vi "UHR-Fleezers Control (fpga) - avogadro 7b enable apd ct.vi"() -> ()   [LabVIEW 2014]
doc: "UHR-Fleezers Instrument Control Code (fpga)"
uses:
  <vilib>/Platform/TimedLoop/XDataNode/timing_clust.ctl
  <vilib>/Platform/TimedLoop/XDataNode/nitl_modes.ctl
  <vilib>/Platform/TimedLoop/XDataNode/wakeup.ctl
  <vilib>/rvi/Emulation/niFpgaGetClockAttributes.vi
  <vilib>/rvi/Emulation/niFpgaSctlEmulationGetInTimedLoop.vi
  <vilib>/rvi/Emulation/niFpgaEmulationReportErrorSimple.vi
  <vilib>/rvi/Emulation/niFpgaProcessEmulError.vi
  <vilib>/rvi/eio/common/nirviEmuTemplateMethod_errors.vi
  <vilib>/rvi/Emulation/niFpgaCriticalErrorInLSC.vi
  <vilib>/rvi/interface/RandomDataEmulation/niFpgaRandomDataHandleErrors.vi
  <vilib>/rvi/Emulation/niFpgaEmulationIsFPGAContextNoSignature.vi
  <vilib>/rvi/errors/niFpgaSetErrorForExecOnDevCompSimple.vi
  <vilib>/rvi/eio/common/nirviEmuReportErrorAndStop.vi
  <vilib>/rvi/DataTransferAndStorage/Container/Common/niFpgaContainerGetUniqueNameForEmu.vi
  <vilib>/rvi/FIFO/Fifo_Resource/nirvififoEmulationSetSize.vi
  <vilib>/rvi/FIFO/Fifo_Resource/nirviFifoEmulationQueueMgr.vi
  <instcachedir>/0/nirviFifoEmulationQueueMgr_E5CAEC123FF24DC58D834DCA3CDAA9B5.lvgen/nirviFifoEmulationQueueMgr_E5CAEC123FF24DC58D834DCA3CDAA9B5_001.vi
  <vilib>/rvi/FIFO/Fifo_Resource/nirvififoEmulationDetermineInputValidOut.vi
  <vilib>/rvi/FIFO/Fifo_Resource/nirvififoEmulationCreateLock.vi
  <vilib>/rvi/FIFO/Fifo_Resource/nirvififoEmulationObtainLock.vi
  <vilib>/rvi/FIFO/Fifo_Resource/nirvififoEmulationReleaseLock.vi
  <vilib>/rvi/occurrence/nirviWaitOnOccurrenceBase.vi
  <vilib>/rvi/errors/nirviReportUnexpectedCaseInternalError.vi
  <vilib>/rvi/errors/nirviReportUnexpectedCaseInternalError (U32).vi
  <vilib>/rvi/DataTransferAndStorage/Container/Common/niFpgaContainerExecOnDevCompGetState.vi
  <vilib>/Utility/error.llb/Clear Errors.vi
  <vilib>/eio/EIONode/EIONode.xnode
  <vilib>/eio/EIOMethodNode/EIOMethodNode.xnode
  <vilib>/rvi/DataTransferAndStorage/Container/XNode/niFpgaContainer.xnode
  <vilib>/rvi/interface/RandomDataEmulation/nirviRandomDataFpgaReadWriteTemplate.vi
  <vilib>/rvi/FIFO/Fifo_Resource/nirvififoEmulationWrite.vi
  <vilib>/rvi/FIFO/Fifo_Resource/niFpgaFifoEmulationRefIn.vi
  <vilib>/addons/control/pid/fpga.llb/XNode/niFpgaPID.xnode
  <vilib>/Platform/TimedLoop/XDataNode/XDataNode.xnode
  <vilib>/rvi/FIFO/Fifo_Resource/nirvififoEmulationRead.vi
  <vilib>/Platform/TimedLoop/XDataNode/XDNodeRunTimeDep.lvlib
  <vilib>/rvi/Memory/Memory_Emulation/niFpgaMemoryEmulationRefIn.vi
panel:
  in  "BD 1 Delay (ticks)":u8
  out "lifetime (ticks)":u16
  in  "Lifetime to FIFO":bool
  in  "Tab Control":T1(tab)=enum."MCL trap control"
  in  "Set 3":bool
  in  "Set 2":bool=TRUE
  in  "Set 1":bool=TRUE
  in  "Trap Pos to FIFO":bool
  in  "N of AI1 Int Acq Sets":i16=2 min=1 max=3 step=1
  out "AI Late Counter":u8
  in  "ai count":u16=400
  in  "+ phase":bool
  in  "Phase count adjustment":i16
  out "Relative phase":i16
  in  "AI to FIFO":bool
  out "BD1 Frequency Out 1":u64
  out "BD1 Frequency Out 2":u64
  out "Trap Pos FIFO Timeout":u16
  out "Trap AI FIFO Timeout":u16
  in  "Trap FIFO Set Timeout":i32
  in  "Tab Control 2":T2(tab)
  in  "Multiple trap 3 position offset \nfile":bool
  in  "Piezo offset Y points":u64
  in  "Piezo offset X points":u64
  in  "Piezo offset Xmin":u64
  in  "Piezo Offset Ymin":u64
  in  "Piezo Offset Increment":u64
  out "BD1 amplitude 1 out":u16
  out "BD1 amplitude 2 out":u16
  in  "FB output range":cluster{"output low":i16, "output high":i16}={"output low"=0, "output high"=3000}
  in  "FB Gains":T3={"proportional gain (Kc)"=10, "integral gain (Kc*Ts/Ti)"=5, "derivative gain (Kc*Td/Ts)"=0}
  in  "RF synth green feedback max":i16=4000
  in  "RD":bool=TRUE
  in  "Swap F1 and F2":bool
  in  "Cont. Scan":bool
  in  "Abort scan":bool
  in  "Cycles per step":u64
  in  "Scan BD":bool
  in  "Number of scans":u16
  in  "Scan steps":u64
  in  "Scan freq.  increment":i64
  out "Scanning":bool
  in  "Start scan":bool
  in  "OSK Bd 1":bool
  in  "Reset Bd 1":bool
  in  "PMODE":bool=TRUE
  in  "Number Interlace Cycles":u8=2 min=1 max=3
  in  "Interlace Off Parameters":u8=1 min=1 max=3
  in  "Interlace ON/OFF":bool
  out "DIO Relative phase":i16
  in  "Phase count adjustment (DIO)":i16
  in  "+ phase (DIO)":bool
  out "DIO Late Counter":u8
  in  "DIO count 1 (ticks)":u16=400
  in  "DIO count 2 (ticks)":u16=400
  in  "DIO count 3 (ticks)":u16=400
  out "AI2 Y Sum Set 2":i16
  out "AI2 Y Sum Set 1":i16
  in  "FB Setpoint Set 1":i16 min=0 step=1
  in  "FB Reset Set 1":bool
  in  "FB On/Off Set 1":bool
  in  "FB Reset Set 2":bool
  in  "FB On/Off Set 2":bool
  in  "FB Setpoint Set 2":i16 min=0 step=1
  out "Scan I":u64
  in  "Amp switch delay":u8=5
  in  "RF synth bd controls green":bool
  in  "Phase Trap 2":fxp<+,14,14>
  in  "Phase Trap 1":fxp<+,14,14>
  in  "Phase offset method":u8
  in  "BD 1 Amplitude 1":u16
  in  "BD 1 Frequency 1":u64
  in  "BD 1 Amplitude 2":u16
  in  "BD 1 Frequency 2":u64
  in  "BD 1 Amplitude 3":u16
  in  "BD 1 Frequency 3":u64
  in  "Next trap write delay (ticks)":u8 caption="Count(Ticks)"
  out "Random phase generated":fxp<+,14,14>
  in  "RF phase reset before cycles":bool
  in  "Ready Write":bool
  in  "Data":i64
  in  "Address 2":u32
  out "Piezo X out":i16
  out "Piezo Y out":i16
  in  "Piezo Trap ON/Off (AO3)":i16
  in  "Piezo Trap X (AO5)":i16
  in  "Piezo Trap Y (AO4)":i16
  in  "Symmetric force feedback\nand raster scan":bool
  in  "FB Min frequency":u64
  in  "FB Max Frequency":u64
  in  "Dynamic Force FB (Ronen)":bool
  in  "Trap pos. FB Range":T4={"FB2 output low"=-1.0, "FB2 output high"=0.999969482421875}
  in  "Trap Pos. FB Gains":T5={"proportional gain (Kc)"=0.999969482421875, "integral gain (Kc*Ts/Ti)"=0.999969482421875, "derivative gain (Kc*Td/Ts)"=0.0}
  in  "B factor":fxp<+/-,32,16>
  in  "Negate Diff?":bool
  in  "Diff FB Measurement?":bool
  in  "FB Trig Integrate":u32=1
  out "TTrig?":bool
  in  "TTrig Negate Pos":bool=TRUE
  out "Trap Pos FB Int Signal":fxp<+/-,24,9> format="%.18g"
  out "Trap Pos FB Int-Norm Signal":fxp<+/-,16,1> format="%.16g"
  in  "FPGA TTrig Thresh":i64
  in  "FPGA Trap Trig":bool
  out "Trap Pos FB Action":i64
  in  "Trap Pos. FB Offset Factor":i64
  in  "Trap Pos. FB Mult Factor":i64=2
  in  "Trap Pos. FB Reset":bool
  in  "Trap Pos FB Monitor T1 or T2":bool
  in  "AI1 X Scale":u16
  in  "Trap Pos FB Int Count":u16=100
  in  "Trap Pos FB Negate Action":bool
  out "AI1 X Set 2":fxp<+/-,16,1>
  out "AI1 X Set 1":fxp<+/-,16,1>
  in  "Trap Pos. FB SP":fxp<+/-,16,1>
  in  "Force feedback":bool
  out "TTrig Sig":i64
  out "TTrig Fin Thresh":i64
  in  "ScanTrap 3 or Fl-laser":bool
  in  "1D or 2D Scan?":bool
  in  "Abort scan (MCL)":bool
  in  "MCL Scan Axis":bool
  in  "Cont. Scan (MCL)":bool
  out "Scan I (MCL)":u64
  in  "Number of scans (MCL)":u16
  out "Scanning MCL":bool
  in  "Scan steps (MCL)":u64
  in  "Cycles per step (MCL)":u64
  in  "Scan freq.  increment (MCL)":i16
  in  "Start scan (MCL)":bool
  in  "AO2 (X)":i16
  in  "AO1 (Y)":i16
  out "MCL Late Counter":u8
  in  "MCL count":u32=800
  out "MCL Relative Phase":i16
  in  "Phase count adjustment (MCL)":i16
  in  "+ phase (MCL)":bool
  in  "Lifetime events to read blue":u16=100
  in  "Lifetime read blue fifo":bool
  out "lifetime events in fifo":u16
  out "APD2 int gate":bool
  out "APD3 out state":bool
  in  "APD Gate Operating Mode":u8 max=2 step=1
  in  "Invert APD Gate":bool
  in  "APD Gate OFF Count":u16=100
  in  "APD Gate ON Count":u16=300
  out "APD 1 Gate Late Counter":u8
  out "APD 1 Gate Relative Phase":i16
  in  "Phase count adjustment (APD 1 Gate)":i16
  in  "+ phase (APD 1 Gate)":bool
  out "APD 2 Counts 0":u32
  out "APD 2 Counts 1":u32
  out "APD 1 Counts 0":u32
  out "APD 1 Counts 1":u32
  out "APD1 out state":bool
  in  "APD AO scale factor":i16=1
  in  "APD to FIFO":bool
  in  "APD Acq Rate Count":u32=20000000
  out "APD Acq Late Counter":u8
  out "APD Acq Relative Phase":i16
  in  "Phase Count Adjustment (APD Acq)":i16
  in  "+ phase (APD Acq)":bool
  in  "Phase count adjustment (APD 2 Gate)":i16
  out "APD 2 Gate Late Counter":u8
  out "APD 2 Gate Relative Phase":i16
  in  "+ phase (APD 2 Gate)":bool
  out "APD2 out state":bool
  out "APD 3 Counts 0":u32
  out "APD 3 Counts 1":u32
  out "APD 3 Gate Late Counter":u8
  in  "Phase count adjustment (APD 3 Gate)":i16
  out "APD 3 Gate Relative Phase":i16
  in  "+ phase (APD 3 Gate)":bool
  out "APD1 int gate":bool
  out "APD3 int gate":bool
  in  "Lifetime timeout APD1":u16=200
  in  "Laser choice 2":u8=100
  in  "Laser choice 1":u8=100
  in  "Laser choice 0":u8=100
  in  "FL interlace OFF count 2":u16=100
  in  "FL interlace OFF count 1":u16=100
  in  "FL interlace ON count 2":u16=300
  in  "Fl interlace ON count 1":u16=300
  in  "D3 2":i16
  in  "I3 2":i16=5
  in  "P3 2":i16=10
  in  "Green FB Setpoint 2":i16=250 min=0 step=1
  in  "Green FB Reset 2":bool
  in  "D3":i16
  in  "I3":i16=5
  in  "P3":i16=10
  in  "Green Filter Flipper":bool
  in  "Green FB Count":u16=1200
  out "Green Late Counter":u8
  out "Green FB Relative Phase":i16
  in  "Phase count adjustment (Green FB)":i16=10
  in  "+ phase (Green FB)":bool
  out "Green FB Sum":i16
  in  "Green int current ON count adj":u16=150
  in  "Current Out":u16=30000
  in  "Green FB On/Off":bool
  in  "Green FB Setpoint":i16=250 min=0 step=1
  in  "Green FB Reset":bool
  in  "Operating Mode 2":u8=2 max=2 step=1
  in  "Invert GI 2":bool
  in  "Green interlace OFF count 2":u16=900
  in  "Green interlace ON count 2":u16=300
  out "GI Late Counter 2":u8
  out "GI Relative phase 2":i16
  in  "Phase count adjustment (GI) 2":i16=20
  in  "+ phase (GI) 2":bool
  in  "FL interlace OFF count 0":u16=100
  out "GI Relative phase":i16
  in  "Phase count adjustment (GI)":i16
  in  "+ phase (GI)":bool
  in  "FL interlace ON count 0":u16=300
  out "GI Late Counter":u8
  in  "Invert GI":bool
  in  "Operating Mode":u8 max=2 step=1
  out "green FB running":bool
  in  "+ phase (RI)":bool
  out "RI Relative phase":i16
  out "RI Late Counter":u8
  in  "Red interlace ON count":u16=300
  in  "Red interlace OFF count":u16=100
  in  "Invert RI":bool
  in  "Red Laser Operating Mode":u8 max=2 step=1
  in  "Phase count adjustment (RI)":i16
  out "Red FB Intensity":i16
  in  "RI Current Out":u16=30000
  in  "Red FB On/Off":bool
  in  "D4":i16
  in  "I4":i16=5
  in  "P4":i16=10
  in  "Red FB Setpoint":i16=250 min=0 step=1
  in  "Red FB Reset":bool
  in  "RI Operating Mode 2":u8=2 max=2 step=1
  in  "Invert RI 2":bool
  in  "Phase count adjustment (BI AO)":i16=20
  in  "Blue current ON count adj (AO)":u16=150
  in  "BI Current Out":i16=30000
  in  "Blue FB On/Off":bool
  in  "D5":i16
  in  "I5":i16=5
  in  "P5":i16=10
  in  "Blue FB Setpoint":i16=250 min=0 step=1
  in  "Blue FB Reset":bool
  in  "BI Operating Mode (AO)":u8=2 max=2 step=1
  in  "Invert BI (AO)":bool
  in  "Blue OFF count (AO)":u16=900
  in  "Blue ON count (AO)":u16=300
  out "BI Late Counter (AO)":u8
  out "BI Relative phase (AO)":i16
  in  "+ phase (BI AO)":bool
  in  "Phase count adjustment (BI D)":i16
  in  "Blue Laser Operating Mode (D)":u8 max=2 step=1
  in  "Invert BI (D)":bool
  in  "Blue interlace OFF count (D)":u16=100
  in  "Blue interlace ON count (D)":u16=300
  out "Blue Late Counter (D)":u8
  out "BI Relative phase (D)":i16
  in  "+ phase (BI D)":bool
  out "Blue Intensity":i16
  in  "Invert EMCCD Gate":bool
  in  "EMCCD Gate ON count":u16=300
  in  "EMCCD Gate OFF count":u16=100
  out "EMCCD Late counter":u8
  out "EMCCD relative phase":i16
  in  "+ phase (EMCCD Gate)":bool
  in  "EMCCD Gate Operating Mode":u8 max=2 step=1
  in  "Phase Count Adjustment EMCCD Gate":i16
  # "Raster Scan AOD"
  # "1 (X)"
  # "2 (Y)"
  # "IR Intensity Feedback (RF BD 1)"
  # "FB Gains Set 1"
  # "FB output range 1"
  # "IR Intensity Feedback (RF BD 2) -\nonly when using BD 2 for green laser AOM (not trap Y)"
  # "Keep below 4096 (12 bits) to stay within range of RF board. Going over doesn't saturate, it truncates higher bits."
  # "RF phase offset control"
  # "Methods are:\n0 - Default, do nothing at all (no phase offset writes)\n1 - Manual phase adjustment\n2 - Cycle the phase adjustment using the input phase numbers as increment values for each cycle"
  # "False is usual, True is external loop method"
  # "Parameters if using the external RF switching loop"
  # "Parameters if using the usual internal RF switching method"
  # "FB Triggering Excitation Laser"
  # "Trap Pos. FB Gains"
  # "Trap Pos. FB Range"
  # "AO1 (Y)"
  # "2D"
  # "Trap 3"
  # "1D"
  # "AO2 (X)"
  # "Fl Laser"
  # "APD AO for aligning"
  # "Detection Loop"
  # "Green fluorescent laser digital gate interlacing loop"
  # "0 Forced ON\n1 Forced OFF\n2 Interlacing"
  # "ALEX settings:"
  # "Controls for usual IA ME controls green AOM"
  # "Controls for RF synth board controls green AOM"
  # "Green FB Gains"
  # "Red fluorescent laser digital gate interlacing loop"
  # "Detection Loop"
  # "0 Forced ON\n1 Forced OFF\n2 Interlacing"
  # "Analog/FB Control Loop\n(Disabled)"
  # "Digital Control Loop"
  # "Blue laser intensity reading"
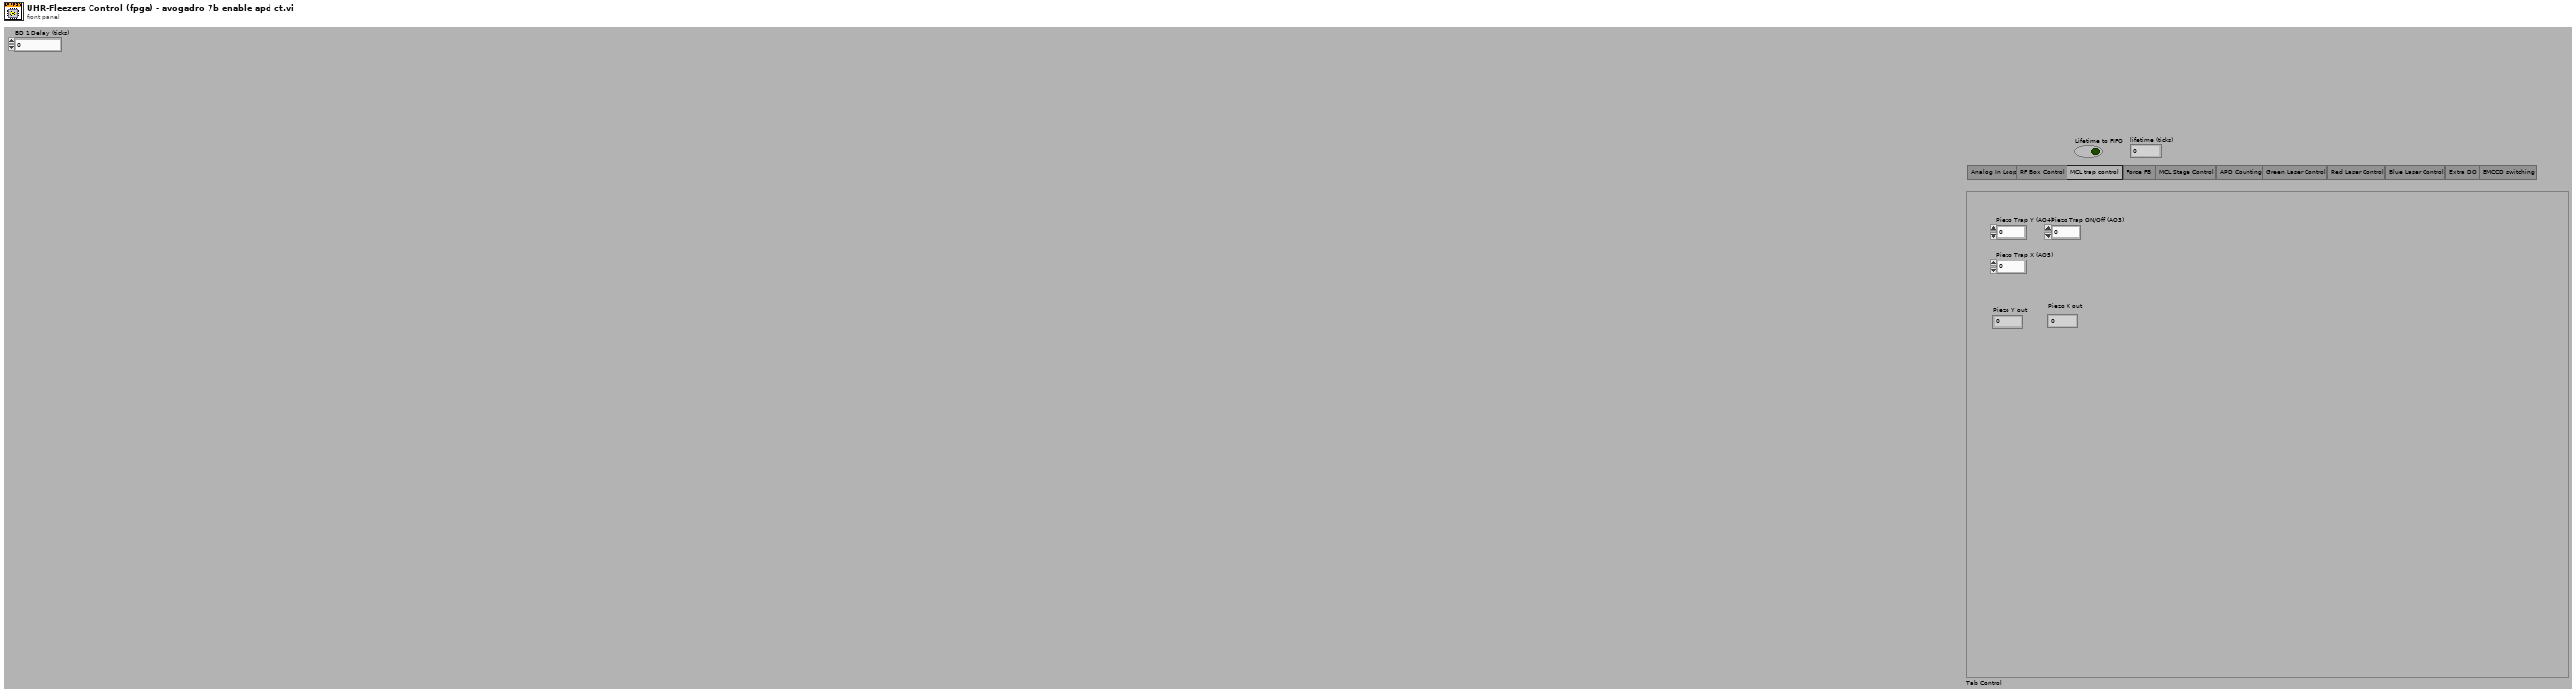
[diagram p1: front panel]
types:
  T1 = enum32{"Analog In Loop", "RF Box Control", "MCL trap control", "Force FB", "MCL Stage Control", "APD Counting", "Green Laser Control", "Red Laser Control", "Blue Laser Control", "Extra DO", "EMCCD switching"}
  T2 = enum32{"Controls", "Interlacing Frequency and Amplitude Values", "Oscillate trap from memory"}
  T3 = cluster{"proportional gain (Kc)":i16, "integral gain (Kc*Ts/Ti)":i16, "derivative gain (Kc*Td/Ts)":i16}
  T4 = cluster{"FB2 output low":fxp<+/-,16,1>, "FB2 output high":fxp<+/-,16,1>}
  T5 = cluster{"proportional gain (Kc)":fxp<+/-,16,1>, "integral gain (Kc*Ts/Ti)":fxp<+/-,16,1>, "derivative gain (Kc*Td/Ts)":fxp<+/-,16,1>}
  T6 = typedef "XDNodeRunTimeDep.lvlib/timing_clust.ctl" = cluster{"Expected End [f-1]":u64, "Actual End [f-1]":u64, "Finished Late? [f-1]":bool, "Expected End [i-1]":u64, "Actual End [i-1]":u64, "Finished Late? [i-1]":bool, "Expected Start [i]":u64, "Actual Start [i]":u64, "Expected Start [f]":u64, "Actual Start [f]":u64, "Source Name":string, "Structure Name":string, "Period":i64, "Deadline":i64, "Offset":i64, "Start":i64, "Priority":i32, "Timeout":i32, "Mode":T7, "Wakeup Reason":T8, "Error":errorcluster, "Source Type":string, "Secondary Source Type":string, "Global End Time":u64, "Global Start Time":u64, "Frame Duration":u64, "Iteration Duration":u64, "Assigned CPU":i32, "I/O Scan Engine Mode":u32}
  T7 = typedef "XDNodeRunTimeDep.lvlib/nitl_modes.ctl" = enum32{"No Change", "Process missed periods, maintain original phase", "Discard missed periods, maintain original phase", "Process missed periods, ignore original phase", "Discard missed periods, ignore original phase"}
  T8 = typedef "XDNodeRunTimeDep.lvlib/wakeup.ctl" = enum32{"Normal", "Aborted", "Asynchronous wakeup", "Timing source error", "Timed loop error", "Timeout"}
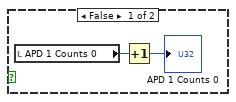
[diagram p3: hidden frame]
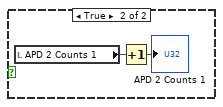
[diagram p5: hidden frame]
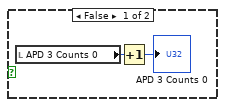
[diagram p7: hidden frame]
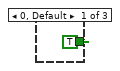
[diagram p8: hidden frame]
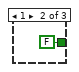
[diagram p9: hidden frame]
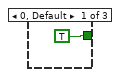
[diagram p10: hidden frame]
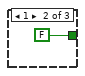
[diagram p11: hidden frame]
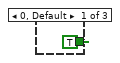
[diagram p12: hidden frame]
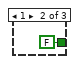
[diagram p13: hidden frame]
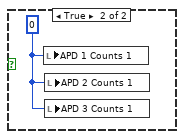
[diagram p14: hidden frame]
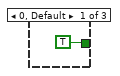
[diagram p16: hidden frame]
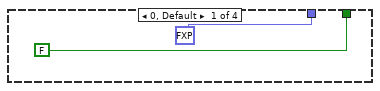
[diagram p18: hidden frame]
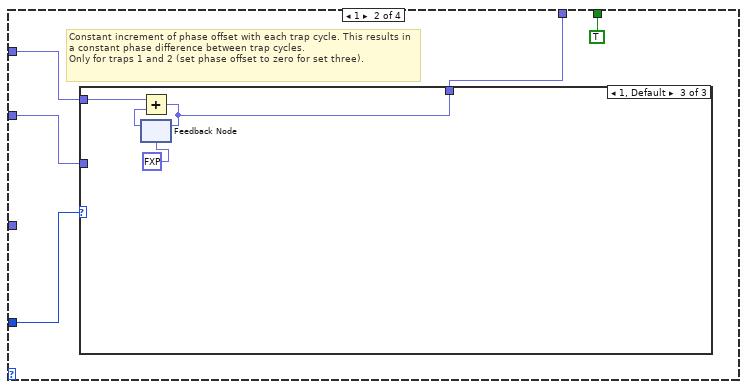
[diagram p19: hidden frame]
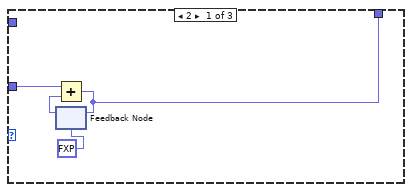
[diagram p20: hidden frame]
diagram:
  w5 = FALSE
  w11 = i16 0
  w15 = FALSE
  # "EMCCD gating"
  # "BD2 amp"
  # "BD1 amp"
  # "BD2 amp"
  # "BD1 amp"
  # "timing array current index"
  # "timing array"
  # "timing counter (phase adjusted here)"
  # "late counter"
  n1 = disable-structure shown="Disabled" {
    frame Disabled {
      w16 = i16 2 items=["UnSet Ready", "ReadWrite", "Wait Ready"]
      n2 = while "Handshake memory transfer for trap oscillation sin wave data" {
        shift-right: [w18] -> _
        shift-left: w16 -> [w19]
        stop <- FALSE stop-if-true
        # "Write"
        n3 = case shown="1" w19 {
          tunnel: [w22 w27 w28] -> w18
          frame 3, Default {
            w20 = i16 2 items=["UnSet Ready", "ReadWrite", "Wait Ready"]
            w21 = i16 1 items=["UnSet Ready", "ReadWrite", "Wait Ready"]
            n4 = Select(t=w21, s="Ready Write", f=w20) -> (s? t:f=w22:i16)
          }
          frame 1 {
            w27 = i16 0 items=["UnSet Ready", "ReadWrite", "Wait Ready"]
            n5 = xnode ("Memory Write")("Address"="Address 2", "Data"="Data", "Memory In"=refnum<k21> "Trap osc memory") -> ()  [unwired: 1 out]
          }
          frame 0 {
            w28 = i16 2 items=["UnSet Ready", "ReadWrite", "Wait Ready"]
            n6 = local write "Ready Write"(FALSE ("Ready Read")) -> ()
          }
        }
      }
    }
    frame Enabled {
    }
  }
  n7 = flat-sequence "FPGA initialization to do before running any of the loops" {
    tunnel: [u16 0 ("DIO count 3 (ticks)")] -> w4
    tunnel: [w34] -> _
    frame #0 {
      # "UDCLK out enable and set low"
      # "WR"
      # "BD 1"
      # "With the RF synth board initialization now done in a separate fpga vi, now when this vi is started, board is already configured and is ready for interlacing. Just need to set WR high and enabled UDCLK as write and set to low.\nbefore setting data and address bits."
      # "Start up expansion chassis early\nto avoid delays later"
      # "Set data and address values to something safe (a correct setting) so any initial WR and udclk flipping doesn't have a chance to mess anything up. Safe would be setting an unused data entry:"
      n8 = xnode "FPGA I/O Method Node"("Enable"=TRUE) -> ("FPGA I/O Out"=w31:refnum<k21>)  [unwired: 1 in]
      n9 = xnode "FPGA I/O Node"("Chassis2/Mod1/AO0"=u16 0 ("Chassis2/Mod4/AO0")) -> ("Chassis2/Mod2/AI0"=w34:i16)  [unwired: 2 in, 2 out]
      n10 = xnode "FPGA I/O Node"("Connector1/DIO15"=TRUE) -> ()  [unwired: 1 in, 1 out]
      n11 = xnode "FPGA I/O Node"("I/O Item"=FALSE ("Connector1/DIO30"), "FPGA I/O In"=w31) -> ()  [unwired: 1 out]
      n12 = xnode "FPGA I/O Node"("Connector1/DIO0"=FALSE, "Connector1/DIO1"=FALSE, "Connector1/DIO2"=FALSE, "Connector1/DIO3"=FALSE, "Connector1/DIO4"=FALSE, "Connector1/DIO5"=FALSE, "Connector1/DIO6"=FALSE, "Connector1/DIO7"=FALSE, "Connector1/DIO8"=FALSE, "Connector1/DIO9"=FALSE, "Connector1/DIO10"=FALSE, "Connector1/DIO11"=FALSE, "Connector1/DIO12"=FALSE, "Connector1/DIO13"=FALSE) -> ()  [unwired: 14 in, 14 out]
    }
  }
  n13 = node-c288() -> (w7:T6)  [unwired: 1 in]
  n14 = timed-loop "RF box board DIO control: control bits" {
    timing: w7 -> [_]
    timing-out: [_] -> w6
    tunnel: [w53] -> _
    tunnel: w4 -> [w53]
    stop <- FALSE stop-if-true
    n15 = xnode "FPGA I/O Node"("Connector1/DIO16"="RD", "Connector1/DIO17"="PMODE", "Connector1/DIO18"="OSK Bd 1", "Connector1/DIO19"="Reset Bd 1", "Connector0/DIO3"="Green Filter Flipper") -> ()  [unwired: 5 in, 5 out]
  }
  n16 = node-c288(w6) -> ()
  n17 = local read "AO1 (Y)"() -> (w13:i16)
  n18 = local read "AO2 (X)"() -> (w12:i16)
  n19 = To Unsigned Long Integer(number=w4) -> (unsigned 32bit integer=w3:u32)
  n20 = disable-structure shown="Disabled" {
    disable-tunnel: w4 -> [w60 _]
    frame Disabled {
      n21 = while "Excitation laser intensity feedback measurement (all lasers)" {
        shift-right: [w61] -> _
        shift-left: w60 -> [w66]
        stop <- FALSE stop-if-true
        n22 = flat-sequence {
          tunnel: w66 -> [w68]
          tunnel: [w69] -> w64
          tunnel: [w68] -> w62
          tunnel: [w75] -> w65
          tunnel: w64 -> [w75]
          tunnel: [w74] -> w63
          tunnel: w62 -> [w74]
          tunnel: [w87] -> w61
          tunnel: w65 -> [w98]
          tunnel: w63 -> [w95]
          frame #0 {
            n23 = call "Loop Timer9"("Count(Ticks)"=w68) -> ("Tick Count(Ticks)"=w69:u16)
          }
          frame #1 {
            # "Design note:\n\nAll lasers need to be measured at the same \ntime because the AI expansion module\ncannot independently time the measurements\nwithin our requirements: there is dead time.\n\nThis probably wouldn't be an issue with the built\nin AI on the fpga board itself."
            n24 = xnode "FPGA I/O Node"("Connector1/DIO35"=TRUE) -> ("Chassis2/Mod1/AI2"=→"Blue Intensity", "Chassis2/Mod1/AI1"=→"Red FB Intensity", "Chassis2/Mod1/AI0"=→"Green FB Sum")  [unwired: 4 in, 4 out]
          }
          frame #2 {
            n25 = feedback-in #1(w98) -> ()
            n26 = feedback #1(w98) -> (w97:u16)
            n27 = Subtract(x=w98, y=w97) -> (x-y=w96:u16)
            n28 = xnode "FPGA I/O Node"("Connector1/DIO35"=FALSE) -> ()  [unwired: 1 in, 1 out]
            n29 = Subtract(x=w96, y=w95) -> (x-y=w77:u16)
            n30 = Subtract(x="Green FB Count", y=w77) -> (x-y=w91:u16)
            n31 = Number To Boolean Array(number=w77) -> (Boolean array=w78:bool[])
            n32 = Or Array Elements(Boolean array=w78) -> (logical OR=w76:bool)
            n33 = Boolean To (0,1)(Boolean="+ phase (Green FB)") -> (0, 1=w89:i16)
            n34 = Boolean To (0,1)(Boolean=w76) -> (0, 1=w83:i16)
            n35 = Multiply(x=w89, y="Phase count adjustment (Green FB)") -> (x*y=w84:i16)
            n36 = Add(x=w91, y=w84) -> (x+y=w87:u16)
            n37 = To Unsigned Byte Integer(number=w83) -> (unsigned 8bit integer=w80:u8)
            n38 = feedback #2(i16 0) -> (w86:i16)
            n39 = Subtract(x=w86, y=w84) -> (x-y=w85:i16)
            "Green FB Relative Phase" <- w85
            n40 = feedback-in #2(w85) -> ()
            n41 = feedback #3(u8 0) -> (w81:u8)
            n42 = Add(x=w80, y=w81) -> (x+y=w79:u8)
            "Green Late Counter" <- w79
            n43 = feedback-in #3(w79) -> ()
          }
        }
      }
    }
    frame Enabled {
    }
  }
  n44 = disable-structure shown="Disabled" {
    disable-tunnel: w4 -> [w99 _]
    frame Disabled {
      w100 = u16 0
      n45 = while "Green and red fluorescent laser interlacing (Current AO to IA 532 nm AOM ME amp)." {
        shift-right: [w180] -> _
        shift-left: w99 -> [w183]
        shift-right: [w177] -> _
        shift-left: w100 -> [w175]
        shift-right: [w174] -> _
        shift-left: w100 -> [w173]
        stop <- FALSE stop-if-true
        n46 = flat-sequence {
          tunnel: w183 -> [w187]
          tunnel: [w188] -> w182
          tunnel: [w187] -> w181
          tunnel: [w186] -> w176
          tunnel: w175 -> [w186]
          tunnel: w173 -> [w185]
          tunnel: [w185] -> w172
          tunnel: [w192] -> w179
          tunnel: w182 -> [w192]
          tunnel: [w191] -> w178
          tunnel: w181 -> [w191]
          tunnel: w176 -> [w190]
          tunnel: w172 -> [w189]
          tunnel: [w220] -> w180
          tunnel: [w236] -> w177
          tunnel: w179 -> [w247]
          tunnel: w178 -> [w244]
          tunnel: [w205] -> w174
          frame #0 {
            n47 = call "Loop Timer10"("Count(Ticks)"=w187) -> ("Tick Count(Ticks)"=w188:u16)
          }
          frame #1 {
            n48 = xnode "FPGA I/O Node"("Chassis2/Mod4/AO0"=w190, "Chassis2/Mod4/AO1"=w189) -> ()  [unwired: 2 in, 2 out]
          }
          frame #2 {
            # "IF RF synth BD does green, never run FB"
            # "ALEX variable is used by APD acquisition loop\nto turn lasers ON/OFF."
            # "Design note:\n\nThese two laser controls are in the same loop\nbecause the expansion current AI cannot separately\ntime the outputs fast enough for us.  Apparently\nit is because of communication time between the\nexpansion card and the fpga.\n\nSo the two analog control signals have the same timing\nand profile, but independent amplitudes to independently\ncontrol the intensity and feedback for each laser."
            n49 = feedback #4(TRUE) -> (w202:bool)
            n50 = Not(x=w202) -> (.not. x?=w203:bool)
            n51 = feedback-in #4(w203) -> ()
            n52 = Subtract(x="Green interlace OFF count 2", y="Green int current ON count adj") -> (x-y=w229:u16)
            n53 = feedback-in #5(w247) -> ()
            n54 = feedback #5(w247) -> (w246:u16)
            n55 = Add(x="Green int current ON count adj", y="Green interlace ON count 2") -> (x+y=w230:u16)
            n56 = Subtract(x=w247, y=w246) -> (x-y=w245:u16)
            n57 = Select(t=w230, s=w203, f=w229) -> (s? t:f=w241:u16)
            n58 = Subtract(x=w245, y=w244) -> (x-y=w213:u16)
            n59 = case shown="2" "RI Operating Mode 2" {
              tunnel: [TRUE FALSE w253] -> w198
              tunnel: w202 -> [_ _ w250]
              frame 0, Default {
              }
              frame 1 {
              }
              frame 2 {
                n60 = Not(x=w250) -> (.not. x?=w252:bool)
                n61 = Select(t=w252, s="Invert RI 2", f=w250) -> (s? t:f=w253:bool)
              }
            }
            n62 = Subtract(x=w241, y=w213) -> (x-y=w224:u16)
            n63 = case shown="2" "Operating Mode 2" {
              tunnel: [TRUE FALSE w287] -> w200
              tunnel: w202 -> [_ _ w284]
              frame 0, Default {
              }
              frame 1 {
              }
              frame 2 {
                n64 = Not(x=w284) -> (.not. x?=w286:bool)
                n65 = Select(t=w286, s="Invert GI 2", f=w284) -> (s? t:f=w287:bool)
              }
            }
            n66 = Number To Boolean Array(number=w213) -> (Boolean array=w214:bool[])
            n67 = Boolean To (0,1)(Boolean="+ phase (GI) 2") -> (0, 1=w226:i16)
            n68 = Or Array Elements(Boolean array=w214) -> (logical OR=w212:bool)
            n69 = local read item#-1() -> (w197)
            n70 = Boolean To (0,1)(Boolean=w212) -> (0, 1=w219:i16)
            n71 = Multiply(x=w226, y="Phase count adjustment (GI) 2") -> (x*y=w222:i16)
            n72 = local read item#-1() -> (w199)
            n73 = local read "RF synth bd controls green"() -> (w194:bool)
            n74 = To Unsigned Byte Integer(number=w219) -> (unsigned 8bit integer=w215:u8)
            n75 = And(x=w197, y=w198) -> (x .and. y?=w196:bool)
            n76 = Add(x=w224, y=w222) -> (x+y=w220:u16)
            n77 = feedback #6(u8 0) -> (w217:u8)
            n78 = Add(x=w215, y=w217) -> (x+y=w216:u8)
            "GI Late Counter 2" <- w216
            n79 = feedback-in #6(w216) -> ()
            n80 = feedback #7(i16 0) -> (w223:i16)
            n81 = Subtract(x=w223, y=w222) -> (x-y=w221:i16)
            "GI Relative phase 2" <- w221
            n82 = feedback-in #7(w221) -> ()
            n83 = And(x=w200, y=w199) -> (x .and. y?=w201:bool)
            n84 = And(x=w201, y="Green FB On/Off") -> (x .and. y?=w231:bool)
            "green FB running" <- w231
            n85 = And(x=w196, y="Red FB On/Off") -> (x .and. y?=w211:bool)
            n86 = Not(x=w194) -> (.not. x?=w193:bool)
            n87 = case shown="True" w211 {
              tunnel: "RI Current Out" -> [w254 _]
              tunnel: [w254 w263] -> w207
              frame False {
              }
              frame True {
                n88 = local read "Red FB Intensity"() -> (w259:i16)
                n89 = Bundle("P4"="P4", "I4"="I4", "D4"="D4") -> (w255:cluster{"P4":i16, "I4":i16, "D4":i16})  [unwired: 1 in]
                n90 = call "Slower PID.vi"("process variable"=w259, "reset?"="Red FB Reset", "setpoint"="Red FB Setpoint", "PID gains (x 2^8)"=w255, "output range"=cluster{"output high":i16, "output low":i16} {"output high"=32767, "output low"=-32768} ("Green FB output range")) -> ("output"=w266:i16)  [unwired: 10 out]
                n91 = To Long Integer(number=w266) -> (32bit integer=w260:i32)
                n92 = Add(x=w260, y=32768) -> (x+y=w262:i32)
                n93 = To Unsigned Word Integer(number=w262) -> (unsigned 16bit integer=w263:u16)
              }
            }
            n94 = And(x=w231, y=w193) -> (x .and. y?=w195:bool)
            n95 = case shown="True" w195 {
              tunnel: "Current Out" -> [w268 w269]
              tunnel: [w268 w269] -> w235
              frame False {
              }
              frame True {
                n96 = disable-structure shown="Disabled" {
                  frame Disabled {
                    n97 = local read "Green FB Sum"() -> (w274:i16)
                    n98 = Bundle("P3"="P3", "I3"="I3", "D3"="D3") -> (w270:cluster{"P3":i16, "I3":i16, "D3":i16})  [unwired: 1 in]
                    n99 = call "Slower PID.vi"("process variable"=w274, "reset?"="Green FB Reset", "setpoint"="Green FB Setpoint", "PID gains (x 2^8)"=w270, "output range"=cluster{"output high":i16, "output low":i16} {"output high"=32767, "output low"=-32768} ("Green FB output range")) -> ("output"=w280:i16)  [unwired: 10 out]
                    n100 = To Long Integer(number=w280) -> (32bit integer=w275:i32)
                    n101 = Add(x=w275, y=32768) -> (x+y=w277:i32)
                    n102 = To Unsigned Word Integer(number=w277) -> ()  [unwired: 1 out]
                  }
                  frame Enabled {
                  }
                }
              }
            }
            n103 = Boolean To (0,1)(Boolean=w196) -> (0, 1=w206:i16)
            n104 = To Unsigned Word Integer(number=w206) -> (unsigned 16bit integer=w208:u16)
            n105 = Boolean To (0,1)(Boolean=w201) -> (0, 1=w237:i16)
            n106 = To Unsigned Word Integer(number=w237) -> (unsigned 16bit integer=w234:u16)
            n107 = Compound Arithmetic op=MULTIPLY(w208, w207) -> (w205:u16)
            n108 = Compound Arithmetic op=MULTIPLY(w234, w235) -> (w236:u16)
          }
        }
      }
      n109 = while "Blue fluorescent laser interlacing (AO control direct to laser)." {
        shift-right: [w107] -> _
        shift-left: w99 -> [w110]
        shift-right: [w104] -> _
        shift-left: i16 0 -> [w102]
        stop <- FALSE stop-if-true
        n110 = flat-sequence {
          tunnel: w110 -> [w113]
          tunnel: [w114] -> w109
          tunnel: [w113] -> w108
          tunnel: [w112] -> w103
          tunnel: w102 -> [w112]
          tunnel: [w117] -> w106
          tunnel: w109 -> [w117]
          tunnel: [w116] -> w105
          tunnel: w108 -> [w116]
          tunnel: w103 -> [w115]
          tunnel: [w127] -> w107
          tunnel: [w143] -> w104
          tunnel: w106 -> [w155]
          tunnel: w105 -> [w152]
          frame #0 {
            n111 = call "Loop Timer13"("Count(Ticks)"=w113) -> ("Tick Count(Ticks)"=w114:u16)
          }
          frame #1 {
            n112 = xnode "FPGA I/O Node"("Connector0/AO3"=w115) -> ()  [unwired: 1 in, 1 out]
          }
          frame #2 {
            n113 = Subtract(x="Blue OFF count (AO)", y="Blue current ON count adj (AO)") -> (x-y=w136:u16)
            n114 = feedback-in #8(w155) -> ()
            n115 = feedback #8(w155) -> (w154:u16)
            n116 = Add(x="Blue current ON count adj (AO)", y="Blue ON count (AO)") -> (x+y=w137:u16)
            n117 = Subtract(x=w155, y=w154) -> (x-y=w153:u16)
            n118 = Subtract(x=w153, y=w152) -> (x-y=w120:u16)
            n119 = Number To Boolean Array(number=w120) -> (Boolean array=w121:bool[])
            n120 = Boolean To (0,1)(Boolean="+ phase (BI AO)") -> (0, 1=w133:i16)
            n121 = Or Array Elements(Boolean array=w121) -> (logical OR=w119:bool)
            n122 = Boolean To (0,1)(Boolean=w119) -> (0, 1=w126:i16)
            n123 = Multiply(x=w133, y="Phase count adjustment (BI AO)") -> (x*y=w129:i16)
            n124 = To Unsigned Byte Integer(number=w126) -> (unsigned 8bit integer=w122:u8)
            n125 = feedback #9(u8 0) -> (w124:u8)
            n126 = Add(x=w122, y=w124) -> (x+y=w123:u8)
            "BI Late Counter (AO)" <- w123
            n127 = feedback-in #9(w123) -> ()
            n128 = feedback #10(i16 0) -> (w130:i16)
            n129 = Subtract(x=w130, y=w129) -> (x-y=w128:i16)
            "BI Relative phase (AO)" <- w128
            n130 = feedback-in #10(w128) -> ()
            n131 = feedback #11(TRUE) -> (w147:bool)
            n132 = case shown="2" "BI Operating Mode (AO)" {
              tunnel: [TRUE FALSE w171] -> w138
              tunnel: w147 -> [_ _ w168]
              frame 0, Default {
              }
              frame 1 {
              }
              frame 2 {
                n133 = Not(x=w168) -> (.not. x?=w170:bool)
                n134 = Select(t=w170, s="Invert BI (AO)", f=w168) -> (s? t:f=w171:bool)
              }
            }
            n135 = And(x=w138, y="Blue FB On/Off") -> (x .and. y?=w139:bool)
            n136 = case shown="True" w139 {
              tunnel: "BI Current Out" -> [w156 _]
              tunnel: [w156 w158] -> w142
              frame False {
              }
              frame True {
                n137 = local read "Blue Intensity"() -> (w157:i16)
                n138 = Bundle("P5"="P5", "I5"="I5", "D5"="D5") -> (w159:cluster{"P5":i16, "I5":i16, "D5":i16})  [unwired: 1 in]
                n139 = call "Slower PID.vi"("process variable"=w157, "reset?"="Blue FB Reset", "setpoint"="Blue FB Setpoint", "PID gains (x 2^8)"=w159, "output range"=cluster{"output high":i16, "output low":i16} {"output high"=32767, "output low"=0} ("Green FB output range")) -> ("output"=w158:i16)  [unwired: 10 out]
              }
            }
            n140 = Not(x=w147) -> (.not. x?=w144:bool)
            n141 = Select(t=w137, s=w144, f=w136) -> (s? t:f=w149:u16)
            n142 = Subtract(x=w149, y=w120) -> (x-y=w131:u16)
            n143 = Add(x=w131, y=w129) -> (x+y=w127:u16)
            n144 = feedback-in #11(w144) -> ()
            n145 = Boolean To (0,1)(Boolean=w138) -> (0, 1=w118:i16)
            n146 = Multiply(x=w118, y=w142) -> (x*y=w143:i16)
          }
        }
      }
    }
    frame Enabled {
    }
  }
  n147 = while "fluorescent laser interlacing (DO)." {
    shift-right: [w294] -> _
    shift-left: w4 -> [w299]
    shift-right: [w293] -> _
    shift-left: w15 -> [w291]
    shift-right: [w290] -> _
    shift-left: u8 0 -> [w288]
    stop <- FALSE stop-if-true
    n148 = flat-sequence {
      tunnel: w299 -> [w303]
      tunnel: [w304] -> w297
      tunnel: [w303] -> w295
      tunnel: [w302] -> w292
      tunnel: w291 -> [w302]
      tunnel: [w301] -> w289
      tunnel: w288 -> [w301]
      tunnel: [w308] -> w298
      tunnel: w297 -> [w308]
      tunnel: [w307] -> w296
      tunnel: w295 -> [w307]
      tunnel: w292 -> [w306]
      tunnel: w289 -> [w305]
      tunnel: [w337] -> w294
      tunnel: w298 -> [w356]
      tunnel: w296 -> [w353]
      tunnel: [w346] -> w293
      tunnel: [w319] -> w290
      frame #0 {
        n149 = call "Loop Timer4"("Count(Ticks)"=w303) -> ("Tick Count(Ticks)"=w304:u16)
      }
      frame #1 {
        n150 = case shown="0, Default" w305 {
          tunnel: w306 -> [w310 w312 w314]
          frame 0, Default {
            w309 = FALSE
            n151 = xnode "FPGA I/O Node"("Connector0/DIO9"=w310, "Connector0/DIO11"=w309, "Connector0/DIO13"=w309) -> ()  [unwired: 3 in, 3 out]
          }
          frame 1 {
            w311 = FALSE
            n152 = xnode "FPGA I/O Node"("Connector0/DIO9"=w311, "Connector0/DIO11"=w312, "Connector0/DIO13"=w311) -> ()  [unwired: 3 in, 3 out]
          }
          frame 2 {
            w313 = FALSE
            n153 = xnode "FPGA I/O Node"("Connector0/DIO9"=w313, "Connector0/DIO11"=w313, "Connector0/DIO13"=w314) -> ()  [unwired: 3 in, 3 out]
          }
        }
      }
      frame #2 {
        # "This lets us alternate interlacing between\nthree different colors\nLaser choice : [0,1,2] = [Blu, Grn, Red]"
        # "Laser counting"
        n154 = feedback-in #12(w356) -> ()
        n155 = feedback #12(w356) -> (w355:u16)
        n156 = Subtract(x=w356, y=w355) -> (x-y=w354:u16)
        n157 = Subtract(x=w354, y=w353) -> (x-y=w315:u16)
        n158 = Number To Boolean Array(number=w315) -> (Boolean array=w331:bool[])
        n159 = Or Array Elements(Boolean array=w331) -> (logical OR=w330:bool)
        n160 = Equal To 0?(x=w315) -> ()  [unwired: 1 out]
        n161 = feedback #13(u8 0) -> (w328:u8)
        n162 = Increment(x=w328) -> (x+1=w325:u8)
        n163 = Less?(x=u8 5, y=w325) -> (x < y?=w326:bool)
        n164 = Select(t=u8 0, s=w326, f=w325) -> (s? t:f=w317:u8)
        n165 = feedback-in #13(w317) -> ()
        n166 = Boolean To (0,1)(Boolean=w330) -> (0, 1=w336:i16)
        n167 = Quotient & Remainder(x=w317, y=u8 2) -> (floor(x/y)=w316:u8)  [unwired: 1 out]
        n168 = To Unsigned Byte Integer(number=w336) -> (unsigned 8bit integer=w333:u8)
        n169 = feedback #14(u8 0) -> (w334:u8)
        n170 = Add(x=w333, y=w334) -> (x+y=w332:u8)
        "GI Late Counter" <- w332
        n171 = feedback-in #14(w332) -> ()
        n172 = Boolean To (0,1)(Boolean="+ phase (GI)") -> (0, 1=w342:i16)
        n173 = Multiply(x=w342, y="Phase count adjustment (GI)") -> (x*y=w339:i16)
        n174 = feedback #15(i16 0) -> (w340:i16)
        n175 = Subtract(x=w340, y=w339) -> (x-y=w338:i16)
        "GI Relative phase" <- w338
        n176 = feedback-in #15(w338) -> ()
        n177 = feedback #16(TRUE) -> (w349:bool)
        n178 = case shown="2" "Operating Mode" {
          tunnel: [TRUE FALSE w446] -> w346
          tunnel: w349 -> [_ _ w443]
          frame 0, Default {
          }
          frame 1 {
          }
          frame 2 {
            n179 = Not(x=w443) -> (.not. x?=w445:bool)
            n180 = Select(t=w445, s="Invert GI", f=w443) -> (s? t:f=w446:bool)
          }
        }
        n181 = Not(x=w349) -> (.not. x?=w345:bool)
        n182 = case shown="0, Default" w316 {
          tunnel: "FL interlace ON count 0" -> [w366 w393 w420]
          tunnel: "FL interlace OFF count 0" -> [w365 w392 w419]
          tunnel: w345 -> [w364 w391 w422]
          tunnel: [w362 w390 w418] -> w343
          tunnel: w315 -> [w363 w394 w421]
          tunnel: "Fl interlace ON count 1" -> [w361 w389 w417]
          tunnel: "FL interlace OFF count 1" -> [w360 w388 w416]
          tunnel: "FL interlace ON count 2" -> [w359 w387 w415]
          tunnel: "FL interlace OFF count 2" -> [w358 w386 w414]
          tunnel: ["Laser choice 0" "Laser choice 1" "Laser choice 2"] -> w319
          frame 0, Default {
            n183 = case shown="1" "Laser choice 0" {
              tunnel: w366 -> [w371 _ _]
              tunnel: w365 -> [w370 _ _]
              tunnel: w364 -> [w369 w375 w381]
              tunnel: w363 -> [w368 w374 w380]
              tunnel: [w367 w373 w379] -> w362
              tunnel: w361 -> [_ w377 _]
              tunnel: w360 -> [_ w376 _]
              tunnel: w359 -> [_ _ w383]
              tunnel: w358 -> [_ _ w382]
              frame 0, Default {
                n184 = Select(t=w371, s=w369, f=w370) -> (s? t:f=w372:u16)
                n185 = Subtract(x=w372, y=w368) -> (x-y=w367:u16)
              }
              frame 1 {
                n186 = Select(t=w377, s=w375, f=w376) -> (s? t:f=w378:u16)
                n187 = Subtract(x=w378, y=w374) -> (x-y=w373:u16)
              }
              frame 2 {
                n188 = Select(t=w383, s=w381, f=w382) -> (s? t:f=w384:u16)
                n189 = Subtract(x=w384, y=w380) -> (x-y=w379:u16)
              }
            }
          }
          frame 1 {
            n190 = case shown="0, Default" "Laser choice 1" {
              tunnel: w393 -> [w399 _ _]
              tunnel: w392 -> [w398 _ _]
              tunnel: w391 -> [w397 w403 w409]
              tunnel: w394 -> [w396 w402 w408]
              tunnel: [w395 w401 w407] -> w390
              tunnel: w389 -> [_ w405 _]
              tunnel: w388 -> [_ w404 _]
              tunnel: w387 -> [_ _ w411]
              tunnel: w386 -> [_ _ w410]
              frame 0, Default {
                n191 = Select(t=w399, s=w397, f=w398) -> (s? t:f=w400:u16)
                n192 = Subtract(x=w400, y=w396) -> (x-y=w395:u16)
              }
              frame 1 {
                n193 = Select(t=w405, s=w403, f=w404) -> (s? t:f=w406:u16)
                n194 = Subtract(x=w406, y=w402) -> (x-y=w401:u16)
              }
              frame 2 {
                n195 = Select(t=w411, s=w409, f=w410) -> (s? t:f=w412:u16)
                n196 = Subtract(x=w412, y=w408) -> (x-y=w407:u16)
              }
            }
          }
          frame 2 {
            n197 = case shown="1" "Laser choice 2" {
              tunnel: w420 -> [w427 _ _]
              tunnel: w419 -> [w426 _ _]
              tunnel: w422 -> [w425 w431 w437]
              tunnel: w421 -> [w424 w430 w436]
              tunnel: [w423 w429 w435] -> w418
              tunnel: w417 -> [_ w433 _]
              tunnel: w416 -> [_ w432 _]
              tunnel: w415 -> [_ _ w439]
              tunnel: w414 -> [_ _ w438]
              frame 0, Default {
                n198 = Select(t=w427, s=w425, f=w426) -> (s? t:f=w428:u16)
                n199 = Subtract(x=w428, y=w424) -> (x-y=w423:u16)
              }
              frame 1 {
                n200 = Select(t=w433, s=w431, f=w432) -> (s? t:f=w434:u16)
                n201 = Subtract(x=w434, y=w430) -> (x-y=w429:u16)
              }
              frame 2 {
                n202 = Select(t=w439, s=w437, f=w438) -> (s? t:f=w440:u16)
                n203 = Subtract(x=w440, y=w436) -> (x-y=w435:u16)
              }
            }
          }
        }
        n204 = Add(x=w343, y=w339) -> (x+y=w337:u16)
        n205 = feedback-in #16(w345) -> ()
      }
    }
  }
  n206 = while "DAQ AI set 1" {
    shift-right: [w447] -> _
    shift-left: w4 -> [w452]
    stop <- FALSE stop-if-true
    n207 = flat-sequence {
      tunnel: w452 -> [w462]
      tunnel: [w463] -> w450
      tunnel: [w462] -> w449
      tunnel: [w473] -> w460
      tunnel: [w472] -> w459
      tunnel: [w471] -> w458
      tunnel: [w470] -> w457
      tunnel: [w469] -> w456
      tunnel: [w468] -> w455
      tunnel: [w467] -> w454
      tunnel: [w466] -> w453
      tunnel: [w465] -> w451
      tunnel: w450 -> [w465]
      tunnel: w449 -> [w464]
      tunnel: [w464] -> w448
      tunnel: [w505] -> w447
      tunnel: w460 -> [w531]
      tunnel: w459 -> [w497]
      tunnel: w458 -> [w498]
      tunnel: w457 -> [w475]
      tunnel: w456 -> [w521]
      tunnel: w455 -> [w520]
      tunnel: w454 -> [w519]
      tunnel: w453 -> [w518]
      tunnel: w451 -> [w515]
      tunnel: w448 -> [w512]
      frame #0 {
        n208 = call "Loop Timer3"("Count(Ticks)"=w462) -> ("Tick Count(Ticks)"=w463:u16)
      }
      frame #1 {
        # "Signal changed to DIO15 to ease\nmeasurement in the room - change\nback for large code"
        n209 = xnode "FPGA I/O Node"("Connector0/DIO15"=TRUE ("Connector1/DIO33")) -> ("Connector0/AI0"=w473:i16, "Connector0/AI1"=w472:i16, "Connector0/AI2"=w471:i16, "Connector0/AI3"=w470:i16, "Connector0/AI4"=w469:i16, "Connector0/AI5"=w468:i16, "Connector0/AI6"=w467:i16, "Connector0/AI7"=w466:i16)  [unwired: 9 in, 9 out]
      }
      frame #2 {
        w501 = FALSE ("AI to FIFO")
        # "Normalize by trap bead QPD sum, AI3"
        # "Adjust phase after data acquired if button pressed"
        n210 = feedback #17(i16 1) -> (w524:i16)
        n211 = Increment(x=w524) -> (x+1=w530:i16)
        n212 = Scale By Power Of 2(n="AI1 X Scale", x=w497) -> (x*2^n=w495:i16)
        n213 = Greater?(x=w530, y="N of AI1 Int Acq Sets") -> (0:w527:bool)
        n214 = Select(t=i16 1, s=w527, f=w530) -> (s? t:f=w529:i16)
        n215 = feedback-in #17(w529) -> ()
        n216 = Divide(x=w495, y=w475) -> (x/y=w494:fxp<+/-,16,1>)
        n217 = feedback #18(w501) -> (w499:bool)
        n218 = feedback #19(w501) -> (w517:bool)
        n219 = case shown="1, Default" w524 {
          tunnel: w498 -> [w556 w563 _]
          tunnel: ["Set 1" "Set 2" "Set 3"] -> w522
          tunnel: ["AI to FIFO" w565 w570] -> w516
          tunnel: w517 -> [_ w565 w570]
          tunnel: ["Trap Pos to FIFO" w564 w569] -> w500
          tunnel: w499 -> [_ w564 w569]
          tunnel: w494 -> [w555 w562 _]
          tunnel: [w554 w560 FALSE] -> w481
          tunnel: [w553 w561 u64 0 ("BD1 Frequency Out 2")] -> w480
          frame 1, Default {
            n220 = local read "BD1 Frequency Out 1"() -> (w553:u64)
            n221 = Compound Arithmetic op=AND("Trap Pos to FIFO", "Set 1", "AI to FIFO") -> (w554:bool)
            "AI2 Y Sum Set 1" <- w556
            "AI1 X Set 1" <- w555
          }
          frame 2 {
            n222 = local read "BD1 Frequency Out 2"() -> (w561:u64)
            n223 = Compound Arithmetic op=AND(w564, "Set 2", w565) -> (w560:bool)
            "AI2 Y Sum Set 2" <- w563
            "AI1 X Set 2" <- w562
          }
          frame 3 {
          }
        }
        n224 = And(x=w522, y=w516) -> (x .and. y?=w523:bool)
        n225 = case shown="True" w523 {
          tunnel: w531 -> [_ w584]
          tunnel: w497 -> [_ w583]
          tunnel: w498 -> [_ w582]
          tunnel: w475 -> [_ w581]
          tunnel: w521 -> [_ w580]
          tunnel: w520 -> [_ w579]
          tunnel: w519 -> [_ w578]
          tunnel: w518 -> [_ w577]
          tunnel: 0 ("DMA buffer timeout") -> [_ w586]
          frame False {
          }
          frame True {
            n226 = Build Array(w584, w583, w582, w581, w580, w579, w578, w577) -> (w585:i16[])
            n227 = for {
              tunnel: w585 -> [w588] mode=indexing
              tunnel: w586 -> [w589]
              tunnel: [w587] -> w575 mode=indexing
              n228 = xnode ("FIFO Write")("Element"=w588, "Timeout"=w589) -> ("Timed Out?"=w587:bool)  [unwired: 1 in, 1 out]
            }
            n229 = Or Array Elements(Boolean array=w575) -> (logical OR=w572:bool)
            n230 = Boolean To (0,1)(Boolean=w572) -> (0, 1=w574:i16)
            n231 = feedback #20(u16 0) -> (w573:u16)
            n232 = Add(x=w574, y=w573) -> (x+y=w571:u16)
            "Trap AI FIFO Timeout" <- w571
            n233 = feedback-in #20(w571) -> ()
          }
        }
        n234 = feedback-in #18(w500) -> ()
        n235 = feedback-in #19(w516) -> ()
        n236 = local read "Piezo X out"() -> (w477:i16)
        n237 = local read "Piezo Y out"() -> (w476:i16)
        n238 = case shown="True" w481 {
          tunnel: w480 -> [_ w539]
          tunnel: [u8 0 w536] -> w479
          tunnel: w477 -> [_ w535]
          tunnel: w476 -> [_ w534]
          frame False {
          }
          frame True {
            n239 = Split Number(x=w539) -> (hi(x)=w540:u32, lo(x)=w541:u32)
            n240 = Split Number(x=w540) -> (lo(x)=w542:u16)  [unwired: 1 out]
            n241 = Split Number(x=w541) -> (hi(x)=w543:u16, lo(x)=w544:u16)
            n242 = Build Array "BD 1 nu Stack"(w542, w543, w544, w535, w534) -> (w538:u16[])
            n243 = for {
              tunnel: w538 -> [w551] mode=indexing
              shift-right: [w547] -> w536
              shift-left: u8 0 -> [w548]
              n244 = xnode ("FIFO Method Node")("Element"=w551, "Timeout"="Trap FIFO Set Timeout") -> ("Timed Out?"=w550:bool)  [unwired: 1 in, 1 out]
              n245 = Boolean To (0,1)(Boolean=w550) -> (0, 1=w549:i16)
              n246 = To Unsigned Byte Integer(number=w549) -> (unsigned 8bit integer=w546:u8)
              n247 = Add(x=w546, y=w548) -> (x+y=w547:u8)
            }
          }
        }
        n248 = To Unsigned Word Integer(number=w479) -> (unsigned 16bit integer=w478:u16)
        n249 = feedback #21(u16 0) -> (w492:u16)
        n250 = Add(x=w478, y=w492) -> (x+y=w491:u16)
        "Trap Pos FIFO Timeout" <- w491
        n251 = feedback-in #21(w491) -> ()
        n252 = feedback-in #22(w515) -> ()
        n253 = feedback #22(w515) -> (w514:u16)
        n254 = Subtract(x=w515, y=w514) -> (x-y=w513:u16)
        n255 = xnode "FPGA I/O Node"("Connector0/DIO15"=FALSE ("Connector1/DIO34")) -> ()  [unwired: 1 in, 1 out]
        n256 = Subtract(x=w513, y=w512) -> (x-y=w483:u16)
        n257 = Boolean To (0,1)(Boolean="+ phase") -> (0, 1=w508:i16)
        n258 = Multiply(x=w508, y="Phase count adjustment") -> (x*y=w502:i16)
        n259 = Subtract(x="ai count", y=w483) -> (x-y=w506:u16)
        n260 = Number To Boolean Array(number=w483) -> (Boolean array=w484:bool[])
        n261 = feedback #23(i16 0) -> (w504:i16)
        n262 = Add(x=w506, y=w502) -> (x+y=w505:u16)
        n263 = Subtract(x=w504, y=w502) -> (x-y=w503:i16)
        "Relative phase" <- w503
        n264 = feedback-in #23(w503) -> ()
        n265 = Or Array Elements(Boolean array=w484) -> (logical OR=w482:bool)
        n266 = Boolean To (0,1)(Boolean=w482) -> (0, 1=w489:i16)
        n267 = To Unsigned Byte Integer(number=w489) -> (unsigned 8bit integer=w486:u8)
        n268 = feedback #24(u8 0) -> (w487:u8)
        n269 = Add(x=w486, y=w487) -> (x+y=w485:u8)
        "AI Late Counter" <- w485
        n270 = feedback-in #24(w485) -> ()
      }
    }
  }
  n271 = while "MCL stage control" {
    shift-right: [w613] -> _
    shift-left: w4 -> [w616]
    shift-right: [w606] -> _
    shift-left: w13 -> [w603]
    shift-right: [w605] -> _
    shift-left: w12 -> [w601]
    shift-right: [w600] -> _
    shift-left: w11 -> [w595]
    shift-right: [w598] -> _
    shift-left: w11 -> [w590]
    shift-right: [w596] -> _
    shift-left: w11 -> [w592]
    stop <- FALSE stop-if-true
    n272 = flat-sequence {
      tunnel: w616 -> [w623]
      tunnel: [w624] -> w612
      tunnel: [w623] -> w610
      tunnel: [w622] -> w604
      tunnel: w603 -> [w622]
      tunnel: [w621] -> w602
      tunnel: w601 -> [w621]
      tunnel: w595 -> [w620]
      tunnel: [w620] -> w594
      tunnel: [w619] -> w593
      tunnel: w592 -> [w619]
      tunnel: [w618] -> w591
      tunnel: w590 -> [w618]
      tunnel: w612 -> [w631]
      tunnel: [w631] -> w611
      tunnel: w610 -> [w630]
      tunnel: [w630] -> w609
      tunnel: w604 -> [w629]
      tunnel: w602 -> [w628]
      tunnel: w594 -> [w627]
      tunnel: w593 -> [w626]
      tunnel: w591 -> [w625]
      tunnel: w611 -> [w645]
      tunnel: w609 -> [w644]
      tunnel: [w645] -> w615
      tunnel: [w644] -> w614
      tunnel: [w643] -> w608
      tunnel: [w642] -> w607
      tunnel: [w634] -> w599
      tunnel: [w632] -> w597
      tunnel: [w752] -> w613
      tunnel: w615 -> [w759]
      tunnel: w614 -> [w756]
      tunnel: w608 -> [w754]
      tunnel: w607 -> [w753]
      tunnel: [w754] -> w606
      tunnel: [w753] -> w605
      tunnel: [w735] -> w600
      tunnel: w599 -> [w735]
      tunnel: [w734] -> w598
      tunnel: w597 -> [w734]
      tunnel: ["Piezo Trap ON/Off (AO3)"] -> w596
      frame #0 {
        n273 = call "Loop Timer5"("Count(Ticks)"=w623) -> ("Tick Count(Ticks)"=w624:u32)
      }
      frame #1 {
        n274 = xnode "FPGA I/O Node"("Connector0/AO1"=w629, "Connector0/AO2"=w628, "Connector0/AO3"=w626, "Connector0/AO4"=w627, "Connector0/AO5"=w625) -> ()  [unwired: 5 in, 5 out]
      }
      frame #2 {
        n275 = local read "Scanning MCL"() -> (w657:bool)
        n276 = Or(x=w657, y="Start scan (MCL)") -> (x .or. y?=w652:bool)
        n277 = Not(x="Abort scan (MCL)") -> (.not. x?=w650:bool)
        n278 = And(x=w650, y=w652) -> (x .and. y?=w649:bool)
        n279 = case "Raster scan" shown="False" w649 {
          tunnel: [w690 w733] -> w654
          tunnel: "Start scan (MCL)" -> [_ w718]
          tunnel: [w690 w694] -> w638
          frame False {
            w690 = i16 0
            n280 = local write "Scanning MCL"(FALSE ("scanning")) -> ()
          }
          frame True {
            w704 = i16 0
            w703 = u64 0
            # "scan incr."
            # "freq. incr. mult."
            # "count steps"
            # "count number of cycles"
            n281 = feedback #25(w703) -> (w730:u64)
            n282 = Select(t=w703, s=w718, f=w730) -> (s? t:f=w732:u64)
            n283 = Increment(x=w732) -> (x+1=w729:u64)
            n284 = Greater?(x="Cycles per step (MCL)", y=w729) -> (0:w713:bool)
            n285 = Select(t=w729, s=w713, f=w703) -> (s? t:f=w728:u64)
            n286 = feedback-in #25(w728) -> ()
            n287 = feedback #26(w703) -> (w727:u64)
            n288 = Select(t=w703, s=w718, f=w727) -> (s? t:f=w722:u64)
            n289 = Increment(x=w722) -> (x+1=w726:u64)
            n290 = Add(x="Scan steps (MCL)", y="Scan steps (MCL)") -> (x+y=w725:u64)
            n291 = Select(t=w722, s=w713, f=w726) -> (s? t:f=w708:u64)
            n292 = Greater?(x=w725, y=w708) -> (0:w707:bool)
            n293 = Select(t=w708, s=w707, f=w703) -> (s? t:f=w723:u64)
            n294 = feedback-in #26(w723) -> ()
            n295 = Equal?(x="Scan steps (MCL)", y=w708) -> (x = y?=w712:bool)
            n296 = Greater?(x="Scan steps (MCL)", y=w722) -> (0:w721:bool)
            n297 = feedback #27(w704) -> (w724:i16)
            n298 = Select(t=w704, s=w718, f=w724) -> (s? t:f=w710:i16)
            n299 = Increment(x=w710) -> (x+1=w720:i16)
            n300 = Decrement(x=w710) -> (x-1=w719:i16)
            n301 = Select(t=w720, s=w721, f=w719) -> (s? t:f=w711:i16)
            n302 = Select(t=w710, s=w712, f=w711) -> (s? t:f=w709:i16)
            n303 = Select(t=w710, s=w713, f=w709) -> (s? t:f=w705:i16)
            n304 = Select(t=w705, s=w707, f=w704) -> (s? t:f=w706:i16)
            n305 = feedback-in #27(w706) -> ()
            n306 = feedback #28(w703) -> (w717:u64)
            n307 = Select(t=w703, s=w718, f=w717) -> (s? t:f=w692:u64)
            n308 = Increment(x=w692) -> (x+1=w714:u64)
            n309 = Select(t=w692, s=w707, f=w714) -> (s? t:f=w693:u64)
            n310 = Greater?(x="Number of scans (MCL)", y=w693) -> (0:w700:bool)
            n311 = Multiply(x="Scan freq.  increment (MCL)", y=w710) -> (x*y=w733:i16)
            n312 = Select(t=TRUE, s="Cont. Scan (MCL)", f=w700) -> (s? t:f=w699:bool)
            "Scanning MCL" <- w699
            n313 = Select(t=w693, s=w699, f=w703) -> (s? t:f=w715:u64)
            n314 = feedback-in #28(w715) -> ()
            n315 = Increment(x=w693) -> (x+1=→"Scan I (MCL)":u64)
            n316 = To Word Integer(number=w692) -> (16bit integer=w695:i16)
            n317 = Multiply(x=w695, y="Scan freq.  increment (MCL)") -> (x*y=w694:i16)
          }
        }
        n318 = case shown="True" "Multiple trap 3 position offset \nfile" {
          tunnel: ["Piezo Trap Y (AO4)" w677] -> w635
          tunnel: ["Piezo Trap X (AO5)" w676] -> w633
          frame False {
          }
          frame True {
            n319 = local read "Scan I"() -> (w688:u64)
            n320 = Decrement(x=w688) -> (x-1=w689:u64)
            n321 = Quotient & Remainder(x=w689, y="Piezo offset Y points") -> (x-y*floor(x/y)=w686:u64, floor(x/y)=w684:u64)
            n322 = Multiply(x=w686, y="Piezo Offset Increment") -> (x*y=w683:u64)
            n323 = Multiply(x="Piezo Offset Increment", y=w684) -> (x*y=w681:u64)
            n324 = Add(x=w681, y="Piezo offset Xmin") -> (x+y=w678:u64)
            n325 = Add(x=w683, y="Piezo Offset Ymin") -> (x+y=w679:u64)
            n326 = To Word Integer(number=w678) -> (16bit integer=w676:i16)
            n327 = To Word Integer(number=w679) -> (16bit integer=w677:i16)
          }
        }
        n328 = Select(t=w638, s="1D or 2D Scan?", f=i16 0) -> (s? t:f=w639:i16)
        n329 = Select(t=w654, s="MCL Scan Axis", f=w639) -> (s? t:f=w655:i16)
        n330 = Select(t=w639, s="MCL Scan Axis", f=w654) -> (s? t:f=w653:i16)
        n331 = case shown="True" "ScanTrap 3 or Fl-laser" {
          tunnel: w655 -> [w665 w667]
          tunnel: w653 -> [w660 w671]
          tunnel: "AO2 (X)" -> [w661 w672]
          tunnel: "AO1 (Y)" -> [w664 w673]
          tunnel: [w663 w673] -> w643
          tunnel: [w662 w672] -> w642
          tunnel: w635 -> [w659 w668]
          tunnel: [w659 w666] -> w634
          tunnel: w633 -> [w658 w670]
          tunnel: [w658 w669] -> w632
          frame False {
            n332 = Add(x=w661, y=w660) -> (x+y=w662:i16)
            n333 = Add(x=w664, y=w665) -> (x+y=w663:i16)
          }
          frame True {
            n334 = Add(x=w668, y=w667) -> (x+y=w666:i16)
            n335 = Add(x=w670, y=w671) -> (x+y=w669:i16)
          }
        }
      }
      frame #3 {
        n336 = feedback-in #29(w759) -> ()
        n337 = feedback #29(w759) -> (w758:u32)
        n338 = Boolean To (0,1)(Boolean="+ phase (MCL)") -> (0, 1=w750:i16)
        n339 = Subtract(x=w759, y=w758) -> (x-y=w757:u32)
        n340 = Multiply(x=w750, y="Phase count adjustment (MCL)") -> (x*y=w746:i16)
        n341 = Subtract(x=w757, y=w756) -> (x-y=w738:u32)
        n342 = Subtract(x="MCL count", y=w738) -> (x-y=w748:u32)
        n343 = feedback #30(i16 0) -> (w747:i16)
        n344 = Subtract(x=w747, y=w746) -> (x-y=w745:i16)
        "MCL Relative Phase" <- w745
        n345 = feedback-in #30(w745) -> ()
        n346 = Number To Boolean Array(number=w738) -> (Boolean array=w739:bool[])
        n347 = Or Array Elements(Boolean array=w739) -> (logical OR=w737:bool)
        n348 = Boolean To (0,1)(Boolean=w737) -> (0, 1=w744:i16)
        n349 = Add(x=w748, y=w746) -> (x+y=w752:u32)
        n350 = To Unsigned Byte Integer(number=w744) -> (unsigned 8bit integer=w741:u8)
        n351 = feedback #31(u8 0) -> (w742:u8)
        n352 = Add(x=w741, y=w742) -> (x+y=w740:u8)
        "MCL Late Counter" <- w740
        n353 = feedback-in #31(w740) -> ()
        "Piezo Y out" <- w735
        "Piezo X out" <- w734
      }
    }
  }
  n354 = while "Trap RF control, main calculations (raster scanning, intensity and position feedback, phase control etc) with primary timing trigger" {
    shift-right: [w777] -> _
    shift-left: w4 -> [w776]
    shift-right: [w775] -> _
    shift-left: FALSE ("Swap F1 and F2") -> [w774]
    shift-right: [w770] -> _
    shift-left: u16 0 ("BD 1 Amplitude 3") -> [w768]
    shift-right: [w767] -> _
    shift-left: u64 0 -> [w766]
    shift-right: [w765] -> _
    shift-left: u64 0 -> [w763]
    shift-right: [w764] -> _
    shift-left: u64 0 -> [w761]
    stop <- FALSE stop-if-true
    n355 = flat-sequence {
      tunnel: w774 -> [w783]
      tunnel: w776 -> [w781]
      tunnel: [w783] -> w773
      tunnel: [w782] -> w772
      tunnel: [w781] -> w771
      tunnel: [w780] -> w769
      tunnel: w768 -> [w780]
      tunnel: [w779] -> w762
      tunnel: w761 -> [w779]
      tunnel: [w796] -> w777
      tunnel: [w795] -> w775
      tunnel: w773 -> [w794]
      tunnel: w772 -> [w793]
      tunnel: w771 -> [w792]
      tunnel: [w791] -> w770
      tunnel: w769 -> [w790]
      tunnel: [w789] -> w767
      tunnel: w766 -> [w788]
      tunnel: [w787] -> w765
      tunnel: [w786] -> w764
      tunnel: w763 -> [w785]
      tunnel: w762 -> [w784]
      frame #0 {
        n356 = call "Loop Timer"("Count(Ticks)"=w781) -> ("Tick Count(Ticks)"=w782:u16)
      }
      frame #1 {
        n357 = flat-sequence {
          tunnel: w794 -> [w802]
          tunnel: w790 -> [w797]
          tunnel: [w846] -> w796
          tunnel: [w858] -> w795
          tunnel: w793 -> [w852]
          tunnel: w792 -> [w849]
          tunnel: [w815] -> w791
          tunnel: [w808] -> w789
          tunnel: w788 -> [w807]
          tunnel: [w806] -> w787
          tunnel: [w805] -> w786
          tunnel: w785 -> [w804]
          tunnel: w784 -> [w803]
          frame #0 {
            w798 = -1 ("Timeout")
            # "Operation when you need a long delay for either X or Y to synchonize AOD light out phase (> ~100 ticks)\nor want shorter trap ON timing. Puts some of the delay timing in parallel with the later computations."
            # "Trigger the external loop by sending the boolean FSK value through a FIFO.\nTiming is precise."
            n358 = Boolean To (0,1)(Boolean=w802) -> (0, 1=w801:i16)
            n359 = To Unsigned Word Integer(number=w801) -> (unsigned 16bit integer=w800:u16)
            n360 = xnode ("FIFO Method Node")("Element"=w800, "Timeout"=w798) -> ("FIFO Out"=w799:refnum<k21>)  [unwired: 1 in, 1 out]
            n361 = xnode ("FIFO Method Node")("Element"=w797, "Timeout"=w798, "FIFO In"=w799) -> ()  [unwired: 2 out]
          }
          frame #1 {
            # "Just counts, wraps around, 8 bit"
            # "Which trap cycle"
            # "Just flips back and forth."
            # "If interlacing is off, this is which cycle to use."
            # "Keep track of trap cycles (trap 1, 2, 3...)"
            # "This is the prior cycle's on time"
            # "increment timing\nindex, reset to 0 if \nend of matrix"
            # "Reset to begginning (1) when number of cycles reached."
            # "timing index"
            # "build byte stacks for writing data\n(must correspond to addresses array constant)"
            # "Timing housekeeping"
            # "Adjust phase if late\n(maintains constant phase relationship between cycles)"
            n362 = feedback #32(u8 0 ("t")) -> (w855:u8)
            n363 = Increment(x=w855) -> (x+1=w882:u8)
            n364 = Increment(x="Number Interlace Cycles") -> (x+1=w877:u8)
            n365 = Equal?(x=w882, y=w877) -> (x = y?=w884:bool)
            n366 = Select(t=u8 1, s=w884, f=w882) -> (s? t:f=w854:u8)
            n367 = feedback-in #32(w854) -> ()
            n368 = Increment(x=w854) -> (x+1=w879:u8)
            n369 = Equal?(x=w879, y=w877) -> (x = y?=w880:bool)
            n370 = Select "This cycle"(t=u8 1, s=w880, f=w879) -> (s? t:f=w876:u8)
            n371 = Select(t=w876, s="Interlace ON/OFF", f="Interlace Off Parameters") -> (s? t:f=w822:u8)
            n372 = feedback-in #33(w852) -> ()
            n373 = feedback #33(w852) -> (w851:u16)
            n374 = Select(t=w854, s="Interlace ON/OFF", f="Interlace Off Parameters") -> (s? t:f=w875:u8)
            n375 = Subtract(x=w852, y=w851) -> (x-y=w850:u16)
            n376 = Subtract "The error"(x=w850, y=w849) -> (x-y=w833:u16)
            n377 = case shown="1, Default" w875 {
              tunnel: ["DIO count 1 (ticks)" "DIO count 2 (ticks)" "DIO count 3 (ticks)"] -> w848
              frame 1, Default {
              }
              frame 2 {
              }
              frame 3 {
              }
            }
            n378 = Number To Boolean Array(number=w833) -> (Boolean array=w834:bool[])
            n379 = Or Array Elements(Boolean array=w834) -> (logical OR=w832:bool)
            n380 = Boolean To (0,1)(Boolean=w832) -> (0, 1=w839:i16)
            n381 = To Unsigned Byte Integer(number=w839) -> (unsigned 8bit integer=w836:u8)
            n382 = feedback #34(u8 0) -> (w837:u8)
            n383 = Add(x=w836, y=w837) -> (x+y=w835:u8)
            "DIO Late Counter" <- w835
            n384 = feedback-in #34(w835) -> ()
            n385 = Subtract(x=w848, y=w833) -> (x-y=w847:u16)
            n386 = local read "green FB running"() -> (w828:bool)
            n387 = And(x=w828, y="RF synth bd controls green") -> (x .and. y?=w827:bool)
            n388 = case shown="2" w822 {
              tunnel: [w992 w1201 "BD 1 Frequency 3"] -> w872
              tunnel: [w989 w1208 "BD 1 Amplitude 3"] -> w815
              tunnel: "FB Gains" -> [w1005 w1211 _]
              tunnel: "FB output range" -> [w1006 w1210 _]
              tunnel: w827 -> [_ _ w1231]
              tunnel: [w992 w1209 w1230] -> w808
              tunnel: w807 -> [w991 w1209 w1230]
              tunnel: [w984 u64 0 u64 0] -> w806
              tunnel: [w985 u64 0 u64 0] -> w805
              tunnel: w804 -> [_ w1205 _]
              tunnel: w803 -> [_ w1204 _]
              frame 1, Default {
                w1020 = fxp<+/-,24,9> 0.0 ("AI1 X Set 2")
                w1014 = u16 0
                # "Changed by RG:\nenables symmetric motion of \ntraps during raster scanning \nand force feedback."
                # "Changed by Ronen - correction \nby PID is now implemented not on \nthe Base BD1 frequency but on the last\nfrequency sent."
                # "Added by Ronen -\nUpper and Lower \nLimits for the FB \ngenerated frequency\nto avoid losing bead \nwhen tether breaks"
                # "Explanation of raster scanning:\n1. Cycles: increment counter by 1 every time interlace cycle returns to trap 1. As long as \n  Cycle per Step is larger than counter, keep incrementing counter and do not change step counter.\n  Once counter is equal to Cycles per step, zero counter and increment step counter.\n2. Steps: Increments up every time cycles counter equals cycles per step. Performs the following:\n- To determine DIRECTION of frequency change:  If ScanstepX2 is EQUAL to step counter (full for-back scan finished)\n   frequency increment is set to zero, AND step counter is set to zero. \n   Otherwise: if no change to step counter (because cycleperstep>cycle counter), then no change to frequency\n   increment. \n   If step counter has changed (cycleperstep=cycle counter), then need to figure out direction of frequency change:\n   if step counter is EQUAL to Scansteps: No change to frequency increment\n   Otherwise: If scan steps > step counter - 1 (forward scan NOT completed): increment frequency by 1\n                       If scan steps equal or smaller than step counter -1 (forward scan completed): increment frequency by -1\n\n3. Scans: Increment scan counter every time step counter equals 2Xscan steps (full for-back scan completed)\n    if number of scans > scan counter: Send TRUE to scanning, continue scan\n    if number of scans = scan counter: Send FALSE to Scanning, Scan finished.\n\n  The wire with the asterik can be used as the index for getting the mirror positions in the offset scan."
                # "This signal integration happens no matter what\nso that correct setpoints can be chosen before \nturning on the FB."
                # "Trap 1"
                n389 = local read "AI1 X Set 2"() -> (w1003:fxp<+/-,16,1>)
                n390 = local read "AI1 X Set 1"() -> (w1017:fxp<+/-,16,1>)
                n391 = local read "Scanning"() -> (w1033:bool)
                n392 = Multiply(x=w1003, y="B factor") -> (x*y=w1001:fxp<+/-,48,17>)
                n393 = Or(x=w1033, y="Start scan") -> (x .or. y?=w1030:bool)
                n394 = case shown="True" "Diff FB Measurement?" {
                  tunnel: w1001 -> [w1058 w1067]
                  tunnel: w1017 -> [w1057 w1068]
                  tunnel: [w1055 w1059] -> w1018
                  frame False {
                    n395 = Select(t=w1057, s="Trap Pos FB Monitor T1 or T2", f=w1058) -> (s? t:f=w1055:fxp<+/-,48,17>)
                  }
                  frame True {
                    n396 = Subtract(x=w1068, y=w1067) -> (x-y=w1060:fxp<+/-,48,17>)
                    n397 = Not(x="Negate Diff?") -> (.not. x?=w1066:bool)
                    n398 = Boolean To (0,1)(Boolean="Negate Diff?") -> (0, 1=w1064:i16)
                    n399 = Boolean To (0,1)(Boolean=w1066) -> (0, 1=w1065:i16)
                    n400 = Negate(x=w1064) -> (-x=w1063:i16)
                    n401 = Add(x=w1063, y=w1065) -> (x+y=w1061:i16)
                    n402 = Multiply(x=w1061, y=w1060) -> (x*y=w1059:fxp<+/-,63,32>)
                  }
                }
                n403 = Not(x="Abort scan") -> (.not. x?=w1028:bool)
                n404 = And(x=w1028, y=w1030) -> (x .and. y?=w1027:bool)
                n405 = case "For raster scanning" shown="False" w1027 {
                  tunnel: [i64 0 w1191] -> w987
                  tunnel: "Start scan" -> [_ w1176]
                  tunnel: [u64 1 w1153] -> w1004
                  frame False {
                    n406 = local write "Scanning"(FALSE ("scanning")) -> ()
                  }
                  frame True {
                    w1160 = i64 0
                    w1159 = u64 0
                    # "scan incr."
                    # "freq. incr. mult."
                    # "count steps"
                    # "count number of cycles"
                    n407 = feedback #35(w1159) -> (w1188:u64)
                    n408 = Select(t=w1159, s=w1176, f=w1188) -> (s? t:f=w1190:u64)
                    n409 = Increment(x=w1190) -> (x+1=w1187:u64)
                    n410 = Greater?(x="Cycles per step", y=w1187) -> (0:w1169:bool)
                    n411 = Select(t=w1187, s=w1169, f=w1159) -> (s? t:f=w1186:u64)
                    n412 = feedback-in #35(w1186) -> ()
                    n413 = feedback #36(w1159) -> (w1185:u64)
                    n414 = Select(t=w1159, s=w1176, f=w1185) -> (s? t:f=w1180:u64)
                    n415 = Increment(x=w1180) -> (x+1=w1184:u64)
                    n416 = Add(x="Scan steps", y="Scan steps") -> (x+y=w1183:u64)
                    n417 = Select(t=w1180, s=w1169, f=w1184) -> (s? t:f=w1164:u64)
                    n418 = Greater?(x=w1183, y=w1164) -> (0:w1163:bool)
                    n419 = Select(t=w1164, s=w1163, f=w1159) -> (s? t:f=w1181:u64)
                    n420 = feedback-in #36(w1181) -> ()
                    n421 = Equal?(x="Scan steps", y=w1164) -> (x = y?=w1168:bool)
                    n422 = Greater?(x="Scan steps", y=w1180) -> (0:w1179:bool)
                    n423 = feedback #37(w1160) -> (w1182:i64)
                    n424 = Select(t=w1160, s=w1176, f=w1182) -> (s? t:f=w1166:i64)
                    n425 = Increment(x=w1166) -> (x+1=w1178:i64)
                    n426 = Decrement(x=w1166) -> (x-1=w1177:i64)
                    n427 = Select(t=w1178, s=w1179, f=w1177) -> (s? t:f=w1167:i64)
                    n428 = Select(t=w1166, s=w1168, f=w1167) -> (s? t:f=w1165:i64)
                    n429 = Select(t=w1166, s=w1169, f=w1165) -> (s? t:f=w1161:i64)
                    n430 = Select(t=w1161, s=w1163, f=w1160) -> (s? t:f=w1162:i64)
                    n431 = feedback-in #37(w1162) -> ()
                    n432 = feedback #38(w1159) -> (w1175:u64)
                    n433 = Select(t=w1159, s=w1176, f=w1175) -> (s? t:f=w1171:u64)
                    n434 = Increment(x=w1171) -> (x+1=w1172:u64)
                    n435 = Select(t=w1171, s=w1163, f=w1172) -> (s? t:f=w1170:u64)
                    n436 = Greater?(x="Number of scans", y=w1170) -> (0:w1156:bool)
                    n437 = Multiply(x="Scan freq.  increment", y=w1166) -> (x*y=w1191:i64)
                    n438 = Select(t=TRUE, s="Cont. Scan", f=w1156) -> (s? t:f=w1155:bool)
                    "Scanning" <- w1155
                    n439 = Select(t=w1170, s=w1155, f=w1159) -> (s? t:f=w1173:u64)
                    n440 = feedback-in #38(w1173) -> ()
                    n441 = Increment(x=w1170) -> (x+1=w1153:u64)
                  }
                }
                "Scan I" <- w1004
                n442 = feedback #39(w1014) -> (w1013:u16)
                n443 = Increment(x=w1013) -> (x+1=w1015:u16)
                n444 = Greater Or Equal?(x=w1015, y="Trap Pos FB Int Count") -> (x >= y?=w990:bool)
                n445 = Select(t=w1014, s=w990, f=w1015) -> (s? t:f=w1016:u16)
                n446 = feedback-in #39(w1016) -> ()
                n447 = feedback #40(w1020) -> (w1019:fxp<+/-,24,9>)
                n448 = Add(x=w1018, y=w1019) -> (x+y=w1012:fxp<+/-,24,9>)
                n449 = case "Trap 1 X intensity feedback" shown="True" "FB On/Off Set 1" {
                  tunnel: "BD 1 Amplitude 1" -> [w1193 _]
                  tunnel: [w1193 w1197] -> w989
                  tunnel: w1006 -> [_ w1194]
                  tunnel: w1005 -> [_ w1195]
                  frame False {
                  }
                  frame True {
                    n450 = local read "AI2 Y Sum Set 1"() -> (w1198:i16)
                    n451 = call "Slower PID.vi"("process variable"=w1198, "reset?"="FB Reset Set 1", "setpoint"="FB Setpoint Set 1", "PID gains (x 2^8)"=w1195, "output range"=w1194) -> ("output"=w1199:i16)  [unwired: 10 out]
                    n452 = To Unsigned Word Integer(number=w1199) -> (unsigned 16bit integer=w1197:u16)
                  }
                }
                "BD1 amplitude 1 out" <- w989
                n453 = Select(t=w1020, s=w990, f=w1012) -> (s? t:f=w1023:fxp<+/-,24,9>)
                n454 = feedback-in #40(w1023) -> ()
                n455 = Divide(x=w1012, y="Trap Pos FB Int Count") -> (x/y=w1007:fxp<+/-,16,1>)
                n456 = feedback #41(fxp<+/-,24,9> 0.0 ("AI1 X Set 2")) -> (w1024:fxp<+/-,24,9>)
                n457 = Select(t=w1012, s=w990, f=w1024) -> (s? t:f=w1025:fxp<+/-,24,9>)
                "Trap Pos FB Int Signal" <- w1025
                n458 = feedback-in #41(w1025) -> ()
                n459 = feedback #42(fxp<+/-,16,1> 0.0 ("Trap Pos FB Int-Norm Signal")) -> (w1009:fxp<+/-,16,1>)
                n460 = Select(t=w1007, s=w990, f=w1009) -> (s? t:f=w1008:fxp<+/-,16,1>)
                "Trap Pos FB Int-Norm Signal" <- w1008
                n461 = feedback-in #42(w1008) -> ()
                n462 = case "For position feedback" shown="True" "Force feedback" {
                  tunnel: [i64 0 w1074] -> w986
                  tunnel: w1007 -> [_ w1071]
                  tunnel: w990 -> [_ w1070]
                  frame False {
                  }
                  frame True {
                    n463 = feedback #43(i64 0) -> (w1073:i64)
                    n464 = case shown="True" w1070 {
                      tunnel: [w1075 w1079] -> w1074
                      tunnel: w1073 -> [w1075 _]
                      tunnel: w1071 -> [_ w1078]
                      frame False {
                      }
                      frame True {
                        n465 = xnode ("PID")("process variable"=w1078, "reset?"="Trap Pos. FB Reset", "setpoint"="Trap Pos. FB SP", "PID gains"="Trap Pos. FB Gains", "output range"="Trap pos. FB Range") -> ("output"=w1088:fxp<+/-,16,1>)
                        n466 = Negate(x=w1088) -> (-x=w1087:fxp<+/-,17,2>)
                        n467 = Select(t=w1087, s="Trap Pos FB Negate Action", f=w1088) -> (s? t:f=w1084:fxp<+/-,17,2>)
                        n468 = Scale By Power Of 2(n=u32 15, x=u32 1) -> (x*2^n=w1081:u32)
                        n469 = Multiply(x=w1084, y=w1081) -> (x*y=w1080:fxp<+/-,17,17>)
                        n470 = To Quad Integer(1:w1080) -> (0:w1092:i64)
                        "Trap Pos FB Action" <- w1092
                        n471 = Multiply(x=w1092, y="Trap Pos. FB Mult Factor") -> (x*y=w1090:i64)
                        n472 = Add(x=w1090, y="Trap Pos. FB Offset Factor") -> (x+y=w1079:i64)
                        n473 = disable-structure shown="Disabled" {
                          disable-tunnel: w1079 -> [w1099 _]
                          frame Disabled {
                            w1103 = u32 0
                            n474 = feedback #44() -> (w1100:i64)  [unwired: 1 in]
                            n475 = Add(x=w1099, y=w1100) -> (x+y=w1097:i64)
                            n476 = feedback #45(w1103) -> (w1105:u32)
                            n477 = Increment(x=w1105) -> (x+1=w1094:u32)
                            n478 = Greater Or Equal?(x=w1094, y="FB Trig Integrate") -> (x >= y?=w1095:bool)
                            n479 = Select(t=i64 0, s=w1095, f=w1097) -> (s? t:f=w1101:i64)
                            n480 = feedback-in #44(w1101) -> ()
                            n481 = Select(t=w1103, s=w1095, f=w1094) -> (s? t:f=w1104:u32)
                            n482 = feedback-in #45(w1104) -> ()
                            n483 = And(x=w1095, y="FPGA Trap Trig") -> (x .and. y?=w1102:bool)
                            n484 = case "Trap FB trigger excitation laser ON" shown="True" w1102 {
                              tunnel: w1097 -> [_ w1109]
                              tunnel: w1094 -> [_ w1107]
                              frame False {
                              }
                              frame True {
                                n485 = Not(x="TTrig Negate Pos") -> (.not. x?=w1116:bool)
                                n486 = Boolean To (0,1)(Boolean="TTrig Negate Pos") -> (0, 1=w1114:i16)
                                n487 = Boolean To (0,1)(Boolean=w1116) -> (0, 1=w1115:i16)
                                n488 = Negate(x=w1114) -> (-x=w1113:i16)
                                n489 = Add(x=w1113, y=w1115) -> (x+y=w1112:i16)
                                n490 = Multiply(x=w1112, y=w1109) -> (x*y=w1111:i64)
                                "TTrig Sig" <- w1111
                                n491 = Multiply(x="FPGA TTrig Thresh", y=w1107) -> (x*y=w1108:i64)
                                "TTrig Fin Thresh" <- w1108
                                n492 = Greater Or Equal?(x=w1111, y=w1108) -> (x >= y?=w1110:bool)
                                n493 = case shown="True" w1110 {
                                frame False {
                                }
                                frame True {
                                w1119 = TRUE ("Green FB On/Off")
                                w1121 = u8 2 ("Operating Mode")
                                n494 = local write "Operating Mode 2"(w1121) -> ()
                                n495 = local write "Operating Mode"(w1121) -> ()
                                n496 = local write "Green FB On/Off"(w1119) -> ()
                                n497 = local write "FPGA Trap Trig"(FALSE ("FPGA Trap Trig")) -> ()
                                "TTrig?" <- w1119
                                }
                                }
                              }
                            }
                          }
                          frame Enabled {
                          }
                        }
                      }
                    }
                    n498 = feedback-in #43(w1074) -> ()
                  }
                }
                n499 = case shown="True" "Symmetric force feedback\nand raster scan" {
                  tunnel: [w1037 w1040] -> w984
                  tunnel: w987 -> [w1037 w1041]
                  tunnel: [w1036 w1038] -> w985
                  tunnel: w986 -> [w1036 w1039]
                  frame False {
                  }
                  frame True {
                    n500 = Scale By Power Of 2(n=i16 -1, x=w1041) -> (x*2^n=w1040:i64)
                    n501 = Scale By Power Of 2(n=i16 -1, x=w1039) -> (x*2^n=w1038:i64)
                  }
                }
                n502 = And(x="Force feedback", y="Dynamic Force FB (Ronen)") -> (x .and. y?=w998:bool)
                n503 = case shown="False" w998 {
                  tunnel: w985 -> [w1046 w1050]
                  tunnel: [w1045 w1049] -> w997
                  tunnel: w991 -> [_ w1048]
                  tunnel: w990 -> [_ w1047]
                  frame False {
                    # "(BD1 Frequency 1)"
                    n504 = Add(x="BD 1 Frequency 1", y=w1046) -> (x+y=w1045:u64)
                  }
                  frame True {
                    n505 = case shown="True" w1047 {
                      tunnel: w1050 -> [_ w1054]
                      tunnel: [w1051 w1053] -> w1049
                      tunnel: w1048 -> [w1051 w1052]
                      frame False {
                      }
                      frame True {
                        n506 = Add(x=w1052, y=w1054) -> (x+y=w1053:u64)
                      }
                    }
                  }
                }
                n507 = Select(t=w984, s="Scan BD", f=u64 0) -> (s? t:f=w996:u64)
                n508 = Add(x=w997, y=w996) -> (x+y=w995:u64)
                n509 = In Range and Coerce(upper limit="FB Max Frequency", x=w995, lower limit="FB Min frequency") -> (coerced(x)=w992:u64)  [unwired: 1 out]
                "BD1 Frequency Out 1" <- w992
              }
              frame 2 {
                # "Trap 2"
                n510 = local read "Symmetric force feedback\nand raster scan"() -> (w1207:bool)
                n511 = case shown="True" w1207 {
                  tunnel: "BD 1 Frequency 2" -> [w1214 w1219]
                  tunnel: [w1214 w1215] -> w1201
                  tunnel: w1205 -> [_ w1218]
                  tunnel: w1204 -> [_ w1216]
                  frame False {
                  }
                  frame True {
                    n512 = Subtract(x=w1219, y=w1218) -> (x-y=w1217:u64)
                    n513 = Subtract(x=w1217, y=w1216) -> (x-y=w1215:u64)
                  }
                }
                "BD1 Frequency Out 2" <- w1201
                n514 = case "Trap 2 X intensity feedback" shown="True" "FB On/Off Set 2" {
                  tunnel: [w1220 w1223] -> w1208
                  tunnel: "BD 1 Amplitude 2" -> [w1220 _]
                  tunnel: w1211 -> [_ w1222]
                  tunnel: w1210 -> [_ w1221]
                  frame False {
                  }
                  frame True {
                    n515 = local read "AI2 Y Sum Set 2"() -> (w1226:i16)
                    n516 = call "Slower PID.vi"("process variable"=w1226, "reset?"="FB Reset Set 2", "setpoint"="FB Setpoint Set 2", "PID gains (x 2^8)"=w1222, "output range"=w1221) -> ("output"=w1224:i16)  [unwired: 10 out]
                    n517 = To Unsigned Word Integer(number=w1224) -> (unsigned 16bit integer=w1223:u16)
                  }
                }
                "BD1 amplitude 2 out" <- w1208
              }
              frame 3 {
                # "Fluorescence period"
                n518 = disable-structure shown="Disabled" {
                  disable-tunnel: [w1239 _] -> _
                  disable-tunnel: w1231 -> [w1238 _]
                  frame Disabled {
                    # "Remember if FB was previously on/off"
                    n519 = feedback #46(FALSE) -> (w1234:bool)
                    n520 = case shown="True" w1238 {
                      tunnel: [w1241 w1257] -> w1239
                      tunnel: [w1241 _] -> w1237
                      tunnel: [FALSE TRUE] -> w1235
                      tunnel: w1234 -> [_ w1242]
                      frame False {
                      }
                      frame True {
                        # "Makes it so first time FB run when turned on, the PID sees the detector intensity from the last time FB was running, rather than something near zero. Especially assuming the setpoint is not changing, this will make the FB more stable when resuming, and not overshoot the turnon intensity."
                        # "FB output range: 0 should be low, full scale is 12 bits.\nBut be careful not to go over, then higher bits just get ignored by RF board, so output will actually jump down and be unstable. Keep it under 4000 to be safe."
                        n521 = local read "Green FB Sum"() -> (w1245:i16)
                        n522 = feedback-in #47(w1245) -> ()
                        n523 = feedback #47(i16 0 ("Green FB Sum")) -> (w1244:i16)
                        n524 = Select(t=w1245, s=w1242, f=w1244) -> (s? t:f=w1243:i16)
                        n525 = Bundle("P3 2"="P3 2", "I3 2"="I3 2", "D3 2"="D3 2") -> (w1256:cluster{"P3 2":i16, "I3 2":i16, "D3 2":i16})  [unwired: 1 in]
                        n526 = Bundle("RF synth green feedback max"="RF synth green feedback max", i16 0) -> (w1248:cluster{"RF synth green feedback max":i16, i16})  [unwired: 1 in]
                        n527 = call "Slower PID.vi"("process variable"=w1243, "reset?"="Green FB Reset 2", "setpoint"="Green FB Setpoint 2", "PID gains (x 2^8)"=w1256, "output range"=w1248) -> ("output"=w1258:i16)  [unwired: 10 out]
                        n528 = To Unsigned Word Integer(number=w1258) -> (unsigned 16bit integer=w1257:u16)
                      }
                    }
                    n529 = feedback-in #46(w1235) -> ()
                  }
                  frame Enabled {
                  }
                }
              }
            }
            n530 = Split Number(x=w872) -> (hi(x)=w871:u32, lo(x)=w870:u32)
            n531 = Boolean To (0,1)(Boolean="+ phase (DIO)") -> (0, 1=w844:i16)
            n532 = Split Number(x=w871) -> (lo(x)=w869:u16)  [unwired: 1 out]
            n533 = Split Number(x=w870) -> (hi(x)=w868:u16, lo(x)=w867:u16)
            n534 = Split Number(x=w869) -> (hi(x)=w866:u8, lo(x)=w865:u8)
            n535 = Split Number(x=w868) -> (hi(x)=w864:u8, lo(x)=w863:u8)
            n536 = Split Number(x=w867) -> (hi(x)=w862:u8, lo(x)=w861:u8)
            n537 = Multiply(x=w844, y="Phase count adjustment (DIO)") -> (x*y=w840:i16)
            n538 = feedback #48(TRUE) -> (w830:bool)
            n539 = Not(x=w830) -> (.not. x?=w829:bool)
            n540 = feedback-in #48(w829) -> ()
            n541 = feedback #49(i16 0) -> (w842:i16)
            n542 = Subtract(x=w842, y=w840) -> (x-y=w841:i16)
            "DIO Relative phase" <- w841
            n543 = feedback-in #49(w841) -> ()
            n544 = Add(x=w847, y=w840) -> (x+y=w846:u16)
            n545 = Build Array "BD 1 nu Stack"(w866, w865, w864, w863, w862, w861) -> (w860:u8[])
            n546 = case "Store in RF board F1 or F2" shown="True" w829 {
              tunnel: [w976 w979] -> w858
              tunnel: [u8 10 u8 4] -> w859
              tunnel: "Swap F1 and F2" -> [w977 w979]
              frame False {
                # "for RF synth controls\ngreen: F1/F2 stay same"
                # "F2 address (hex)"
                n547 = Not(x=w977) -> (.not. x?=w976:bool)
              }
              frame True {
                # "low chooses F1"
                # "F1 address (hex)"
              }
            }
            n548 = flat-sequence "Update trap RF synth board settings to be used for the upcoming trap cycle." {
              tunnel: w860 -> [w939]
              tunnel: [w939] -> w825
              tunnel: w859 -> [w940]
              tunnel: w825 -> [w941]
              tunnel: w816 -> [w950]
              tunnel: w817 -> [w949]
              frame #0 {
                # "To possibly delay\nthese writes to very\nend of loop (for x and\ny phase adjust)"
                n549 = call "Wait8"("Count(Ticks)"="Next trap write delay (ticks)") -> ()  [unwired: 1 out]
              }
              frame #1 {
                # "Next trap RF frequency:\n\nWrite next trap cycle frequency to buffer."
                n550 = for {
                  tunnel: w941 -> [w946] mode=indexing
                  tunnel: w940 -> [w944]
                  i -> [w945]
                  n551 = To Unsigned Byte Integer(number=w945) -> (unsigned 8bit integer=w942:u8)
                  n552 = Add(x=w944, y=w942) -> (x+y=w943:u8)
                  n553 = call "Write to RF Synth Bd1 Only.vi"("Address Byte"=w943, "BD 1 Byte"=w946) -> ()  [unwired: 1 in]
                }
              }
              frame #2 {
                # "Send udclk high\n(BD 1 and 2) to make the new frequency active in F1 or F2 word. But it won't actually be the used frequency until FSK switches to it (begining of next cycle)."
                n554 = xnode "FPGA I/O Node"("Connector1/DIO30"=TRUE ("Connector1/DIO15")) -> ()  [unwired: 1 in, 1 out]
              }
              frame #3 {
                n555 = xnode "FPGA I/O Node"("Connector1/DIO30"=FALSE ("Connector1/DIO15")) -> ()  [unwired: 1 in, 1 out]
              }
              frame #4 {
                # "Next trap RF phase offset:\n\nSet the next trap cycle amplitude to the buffer. Won't become active until udclk is set high at proper time at the begining of the next cycle."
                n556 = case shown="True" w950 {
                  tunnel: w949 -> [_ w951]
                  frame False {
                  }
                  frame True {
                    # "phase 1 address start"
                    n557 = for {
                      tunnel: w951 -> [w957] mode=indexing
                      tunnel: u8 0 -> [w955]
                      i -> [w956]
                      n558 = To Unsigned Byte Integer(number=w956) -> (unsigned 8bit integer=w953:u8)
                      n559 = Add(x=w955, y=w953) -> (x+y=w954:u8)
                      n560 = call "Write to RF Synth Bd1 Only.vi"("Address Byte"=w954, "BD 1 Byte"=w957) -> ()  [unwired: 1 in]
                    }
                  }
                }
              }
              frame #5 {
                # "Prep to reset RF phase to zero at start of next cycle. Only reset BD 1. Do nothing to BD 2. This puts the settings in the buffer. A udclk high will make both this phase reset and possibly a new phase offset setting active."
                n561 = case shown="True" "RF phase reset before cycles" {
                  frame False {
                  }
                  frame True {
                    w960 = u8 66  # BD 1 reset
                    n562 = call "write to RF synth bd.vi"("Address Byte"=u8 31, "BD 2 Byte"=u8 2, "BD 1 Byte"=w960) -> ()
                  }
                }
              }
              frame #6 {
                # "Address"
                # "Data BD 1"
                # "If phase reset wasn't chosen previously, these actions will have no affect. For both BD's, data should be binary 10, and address should be hex 1F (bin 01 1111)"
                # "This sets up the digital communication lines to restart phase accumulation (start RF running agin). It cancels out the possible phase reset. Just need to set WR DIO low then udclk DIOhigh  to make this happen. Doing this here early (and not using the usual board write function) speeds things up.\n\nRestarts RF (BD 1 only, BD2 never stopped in first place)."
                n563 = xnode "FPGA I/O Node"("Connector1/DIO0"=FALSE, "Connector1/DIO1"=FALSE, "Connector1/DIO2"=FALSE, "Connector1/DIO3"=FALSE, "Connector1/DIO4"=FALSE, "Connector1/DIO5"=FALSE, "Connector1/DIO6"=TRUE, "Connector1/DIO7"=FALSE, "Connector1/DIO8"=FALSE, "Connector1/DIO9"=TRUE, "Connector1/DIO10"=TRUE, "Connector1/DIO11"=TRUE, "Connector1/DIO12"=TRUE, "Connector1/DIO13"=TRUE) -> ()  [unwired: 14 in, 14 out]
              }
            }
            n564 = feedback #50(fxp<+,8,8> 0.0) -> (w813:fxp<+,8,8>)
            n565 = Increment(x=w813) -> (x+1=w811:fxp<+,8,8>)
            n566 = feedback-in #50(w811) -> ()
            n567 = case "Trap RF phase offset control methods" shown="3" "Phase offset method" {
              tunnel: [fxp<+,14,14> 0.0 ("Phase BD 1") w889 w904 w933] -> w818
              tunnel: "Phase Trap 1" -> [_ w890 w905 _]
              tunnel: w822 -> [_ w891 w906 w934]
              tunnel: [FALSE TRUE TRUE TRUE] -> w816
              tunnel: "Phase Trap 2" -> [_ w887 w902 _]
              tunnel: w811 -> [_ _ w901 _]
              frame 0, Default {
              }
              frame 1 {
                # "Constant increment of phase offset with each trap cycle. This results in a constant phase difference between trap cycles. \nOnly for traps 1 and 2 (set phase offset to zero for set three)."
                n568 = case shown="1, Default" w891 {
                  tunnel: w890 -> [_ _ w897]
                  tunnel: [w893 fxp<+,14,14> 0.0 w898] -> w889
                  tunnel: w887 -> [w892 _ _]
                  frame 2 {
                    n569 = feedback #51(fxp<+,14,14> 0.0) -> (w895:fxp<+,14,14>)
                    n570 = Add(x=w892, y=w895) -> (x+y=w893:fxp<+,14,14>)
                    n571 = feedback-in #51(w893) -> ()
                  }
                  frame 3 {
                  }
                  frame 1, Default {
                    n572 = feedback #52(fxp<+,14,14> 0.0) -> (w900:fxp<+,14,14>)
                    n573 = Add(x=w897, y=w900) -> (x+y=w898:fxp<+,14,14>)
                    n574 = feedback-in #52(w898) -> ()
                  }
                }
              }
              frame 2 {
                # "Changing increment of phase offset with each trap cycle. This results in a constant change in phase difference between trap cycles. \nOnly for traps 1 and 2 (set phase offset to zero for set three)."
                n575 = case shown="2" w906 {
                  tunnel: w905 -> [_ _ w916]
                  tunnel: [w907 fxp<+,14,14> 0.0 w914] -> w904
                  tunnel: w902 -> [w909 _ _]
                  tunnel: w901 -> [w910 _ w917]
                  frame 2 {
                    n576 = Multiply(x=w909, y=w910) -> (x*y=w908:fxp<+,16,16>)
                    n577 = feedback #53(fxp<+,14,14> 0.0) -> (w912:fxp<+,14,14>)
                    n578 = Add(x=w908, y=w912) -> (x+y=w907:fxp<+,14,14>)
                    n579 = feedback-in #53(w907) -> ()
                  }
                  frame 3 {
                  }
                  frame 1, Default {
                    n580 = Multiply(x=w916, y=w917) -> (x*y=w915:fxp<+,16,16>)
                    n581 = feedback #54(fxp<+,14,14> 0.0) -> (w919:fxp<+,14,14>)
                    n582 = Add(x=w915, y=w919) -> (x+y=w914:fxp<+,14,14>)
                    n583 = feedback-in #54(w914) -> ()
                  }
                }
              }
              frame 3 {
                w926 = u32 1013904223  # LCG constant C (add)
                w928 = fxp<+,21,21> 1664525.0  # LCG constant A (multiply)
                # "Set a random phase offset. Random number generated using the LCG method. Constants and method taken from NI white noise generator code (method is general though)."
                # "shift to 14 significant bits"
                n584 = feedback #55(u32 4294967295 ("seed")) -> (w923:u32)
                n585 = Multiply(x=w923, y=w928) -> (x*y=w927:u32)
                n586 = Split Number(x=w923) -> (hi(x)=w929:u16)  [unwired: 1 out]
                n587 = To Unsigned Word Integer(number=w929) -> (unsigned 16bit integer=w921:u16)
                n588 = Add(x=w927, y=w926) -> (x+y=w925:fxp<+,32,32>)
                n589 = To Unsigned Long Integer(number=w925) -> (unsigned 32bit integer=w922:u32)
                n590 = feedback-in #55(w922) -> ()
                n591 = Scale By Power Of 2(n=i8 -2 ("Uniform scale factor"), x=w921) -> (x*2^n=w930:u16)
                n592 = To Fixed-Point(number=w930) -> (fixed-point=w920:fxp<+,14,14>)  [unwired: 1 in]
                "Random phase generated" <- w920
                n593 = case shown="1, Default" w934 {
                  tunnel: [w935 fxp<+,14,14> 0.0 w937] -> w933
                  tunnel: w920 -> [w935 _ w937]
                  frame 2 {
                  }
                  frame 3 {
                  }
                  frame 1, Default {
                  }
                }
              }
            }
            n594 = To Unsigned Word Integer(number=w818) -> (unsigned 16bit integer=w821:u16)
            n595 = Split Number(x=w821) -> (hi(x)=w819:u8, lo(x)=w820:u8)
            n596 = Build Array ("BD 1 A Stack")(w819, w820) -> (w817:u8[])
          }
        }
      }
    }
  }
  n597 = while "APD 2 Counter" {
    tunnel: w4 -> [_]
    stop <- FALSE stop-if-true
    n598 = flat-sequence {
      frame #0 {
        n599 = xnode "FPGA I/O Method Node"("FPGA I/O In"=refnum<k21> "Connector0/DIO8" ("APD 2 DO"), "Timeout"=-1) -> ()  [unwired: 2 out]
      }
      frame #1 {
        n600 = local read "APD2 int gate"() -> (w1262:bool)
        n601 = case shown="True" w1262 {
          frame False {
          }
          frame True {
            n602 = local read "APD2 out state"() -> (w1263:bool)
            n603 = case shown="False" w1263 {
              frame False {
                n604 = local read "APD 2 Counts 0"() -> (w1265:u32)
                n605 = Increment(x=w1265) -> (x+1=→"APD 2 Counts 0":u32)
              }
              frame True {
                n606 = local read "APD 2 Counts 1"() -> (w1267:u32)
                n607 = Increment(x=w1267) -> (x+1=→"APD 2 Counts 1":u32)
              }
            }
          }
        }
      }
    }
  }
  n608 = while "APD 1 Counter" {
    tunnel: w4 -> [_]
    stop <- FALSE stop-if-true
    n609 = flat-sequence {
      frame #0 {
        n610 = xnode "FPGA I/O Method Node"("FPGA I/O In"=refnum<k21> "Connector0/DIO4" ("APD 1 DO"), "Timeout"=-1) -> ()  [unwired: 2 out]
      }
      frame #1 {
        n611 = local read "APD1 int gate"() -> (w1271:bool)
        n612 = case shown="True" w1271 {
          frame False {
          }
          frame True {
            n613 = local read "APD1 out state"() -> (w1272:bool)
            n614 = case shown="True" w1272 {
              frame False {
                n615 = local read "APD 1 Counts 0"() -> (w1274:u32)
                n616 = Increment(x=w1274) -> (x+1=→"APD 1 Counts 0":u32)
              }
              frame True {
                n617 = local read "APD 1 Counts 1"() -> (w1276:u32)
                n618 = Increment(x=w1276) -> (x+1=→"APD 1 Counts 1":u32)
              }
            }
          }
        }
      }
    }
  }
  n619 = while "RF synth board interlacing timing loop" {
    tunnel: w4 -> [_]
    stop <- FALSE stop-if-true
    # "This loop is stalled until the RF FIFO get a value. With this method we gain additional delay time (because  we allow the rest of the main RF loop to procede while this loop waits to send the switch signals - a form of parallelism). This helps to simplify the main RF code. \n\nThe code also allow optimal interlacing while also controlling trap RF phase. \n\nNote: a lot of work has gone into optimizing these methods and it is unclear how they can be made any faster or better than this (many failed tries). Right now there is essentially ~4 ticks (~90 ns ns) of imperfection in the switching from trap 1 to trap 2. ~2 ticks of no RF (phase reset) then ~2 ticks of trap 2 with the wrong amplitude (T1 amplitude). The total ticks is 200, so not a big error.\n\nPhase can be precisely set for each trap. Phase reset and switching, has similar delays as fsk frequency switching. And phase reset and phase offset changes are also not simultaneous. So we can't perfectly line everything up.\n\nIf you start from amp zero though (as for trap 1), the on switch is perfect. Likewise the off is perfect for trap 2. \n\nThe green laser switching is also perfect because of its reduced duty cycle and delays in fsk switching between 80 and 0 MHz."
    n620 = xnode ("FIFO Read")("Timeout"=-1) -> ("Element"=w1303:u16, "FIFO Out"=w1300:refnum<k21>)  [unwired: 1 in, 1 out]
    n621 = Equal To 0?(x=w1303) -> (x = 0?=w1301:bool)
    n622 = Not(x=w1301) -> (.not. x?=w1277:bool)
    n623 = flat-sequence "BD 1 and 2 RF phase and amplitude switching" {
      tunnel: w1277 -> [_]
      tunnel: w1295 -> [w1361]
      tunnel: w1294 -> [w1360]
      tunnel: w1293 -> [w1359]
      tunnel: w1292 -> [w1358]
      tunnel: w1291 -> [w1357]
      tunnel: w1290 -> [w1356]
      tunnel: w1289 -> [w1355]
      tunnel: w1288 -> [w1354]
      tunnel: w1287 -> [w1377]
      tunnel: w1286 -> [w1376]
      tunnel: w1285 -> [w1375]
      tunnel: w1284 -> [w1374]
      tunnel: w1283 -> [w1373]
      tunnel: w1282 -> [w1372]
      tunnel: w1281 -> [w1371]
      tunnel: w1280 -> [w1370]
      frame #0 {
        # "Delay to align amp/frequency switching depending on the method used.\n\nCan also give enough time to do the parallel amplitude calculations"
        n624 = call "Wait"("Count(Ticks)"="Amp switch delay") -> ()  [unwired: 1 out]
      }
      frame #1 {
        # "make phase offset and phase reset active with buffer transfer"
        n625 = xnode "FPGA I/O Node"("Connector1/DIO30"=TRUE) -> ()  [unwired: 1 in, 1 out]
      }
      frame #2 {
        w1351 = FALSE ("Connector1/DIO14")
        # "write phase restart to buffer and reset udclk"
        n626 = xnode "FPGA I/O Node"("Connector1/DIO30"=w1351, "Connector1/DIO15"=w1351) -> ()  [unwired: 2 in, 2 out]
      }
      frame #3 {
        w1352 = TRUE ("Connector1/DIO15")
        # "make phase restart active"
        # "reset WR"
        n627 = xnode "FPGA I/O Node"("Connector1/DIO15"=w1352, "Connector1/DIO30"=w1352) -> ()  [unwired: 2 in, 2 out]
      }
      frame #4 {
        # "Address"
        # "set amp byte 1, and reset udclk"
        n628 = xnode "FPGA I/O Node"("Connector1/DIO0"=w1361, "Connector1/DIO1"=w1360, "Connector1/DIO2"=w1359, "Connector1/DIO3"=w1358, "Connector1/DIO4"=w1357, "Connector1/DIO5"=w1356, "Connector1/DIO6"=w1355, "Connector1/DIO7"=w1354, "Connector1/DIO8"=TRUE, "Connector1/DIO9"=FALSE, "Connector1/DIO10"=FALSE, "Connector1/DIO11"=FALSE, "Connector1/DIO12"=FALSE, "Connector1/DIO13"=TRUE, "Connector1/DIO30"=FALSE) -> ()  [unwired: 15 in, 15 out]
      }
      frame #5 {
        # "write amp byte 1 to buffer"
        n629 = xnode "FPGA I/O Node"("Connector1/DIO15"=FALSE ("Connector1/DIO14")) -> ()  [unwired: 1 in, 1 out]
      }
      frame #6 {
        # "reset WR"
        n630 = xnode "FPGA I/O Node"("Connector1/DIO15"=TRUE) -> ()  [unwired: 1 in, 1 out]
      }
      frame #7 {
        # "Address"
        # "set amp byte 2"
        n631 = xnode "FPGA I/O Node"("Connector1/DIO0"=w1377, "Connector1/DIO1"=w1376, "Connector1/DIO2"=w1375, "Connector1/DIO3"=w1374, "Connector1/DIO4"=w1373, "Connector1/DIO5"=w1372, "Connector1/DIO6"=w1371, "Connector1/DIO7"=w1370, "Connector1/DIO8"=TRUE, "Connector1/DIO9"=FALSE, "Connector1/DIO10"=FALSE, "Connector1/DIO11"=FALSE, "Connector1/DIO12"=TRUE, "Connector1/DIO13"=FALSE) -> ()  [unwired: 14 in, 14 out]
      }
      frame #8 {
        # "write amp byte 2"
        n632 = xnode "FPGA I/O Node"("Connector1/DIO15"=FALSE ("Connector1/DIO14")) -> ()  [unwired: 1 in, 1 out]
      }
      frame #9 {
        w1385 = TRUE ("Connector1/DIO14")
        # "transfer amp bytes 1 and 2 and reset WR"
        n633 = xnode "FPGA I/O Node"("Connector1/DIO30"=w1385, "Connector1/DIO15"=w1385) -> ()  [unwired: 2 in, 2 out]
      }
      frame #10 {
        # "reset udclk"
        n634 = xnode "FPGA I/O Node"("Connector1/DIO30"=FALSE ("Connector1/DIO14")) -> ()  [unwired: 1 in, 1 out]
      }
    }
    n635 = flat-sequence "FSK BD 1 (trap X)" {
      tunnel: w1277 -> [w1305]
      tunnel: [w1305] -> w1279
      tunnel: w1279 -> [w1306]
      frame #0 {
        n636 = call "Wait2"("Count(Ticks)"="BD 1 Delay (ticks)") -> ()  [unwired: 1 out]
      }
      frame #1 {
        # "switch frequency"
        n637 = xnode "FPGA I/O Node"("Connector1/DIO36"=w1306) -> ()  [unwired: 1 in, 1 out]
      }
    }
    n638 = xnode ("FIFO Read")("Timeout"=-1, "FIFO In"=w1300) -> ("Element"=w1296:u16)  [unwired: 2 out]
    n639 = node-c288() -> (w1298:T6)  [unwired: 1 in]
    n640 = timed-loop "Convert amplitude words to bits" {
      timing: w1298 -> [_]
      timing-out: [_] -> w1297
      tunnel: w1296 -> [w1335]
      tunnel: [w1323] -> w1295
      tunnel: [w1322] -> w1294
      tunnel: [w1321] -> w1293
      tunnel: [w1320] -> w1292
      tunnel: [w1319] -> w1291
      tunnel: [w1318] -> w1290
      tunnel: [w1317] -> w1289
      tunnel: [w1316] -> w1288
      tunnel: [w1315] -> w1287
      tunnel: [w1314] -> w1286
      tunnel: [w1313] -> w1285
      tunnel: [w1312] -> w1284
      tunnel: [w1311] -> w1283
      tunnel: [w1310] -> w1282
      tunnel: [w1309] -> w1281
      tunnel: [w1308] -> w1280
      stop <- TRUE stop-if-true
      # "Board 1 Data"
      # "Board 1 Data"
      n641 = Split Number(x=w1335) -> (hi(x)=w1334:u8, lo(x)=w1324:u8)
      n642 = Number To Boolean Array(number=w1334) -> (Boolean array=w1344:bool[])
      n643 = Index Array(array=w1344, index=7) -> (element=w1323:bool)
      n644 = Index Array(array=w1344, index=6) -> (element=w1322:bool)
      n645 = Index Array(array=w1344, index=5) -> (element=w1321:bool)
      n646 = Index Array(array=w1344, index=4) -> (element=w1320:bool)
      n647 = Index Array(array=w1344, index=3) -> (element=w1319:bool)
      n648 = Index Array(array=w1344, index=2) -> (element=w1318:bool)
      n649 = Index Array(array=w1344, index=1) -> (element=w1317:bool)
      n650 = Index Array(array=w1344, index=0) -> (element=w1316:bool)
      n651 = Number To Boolean Array(number=w1324) -> (Boolean array=w1333:bool[])
      n652 = Index Array(array=w1333, index=7) -> (element=w1315:bool)
      n653 = Index Array(array=w1333, index=6) -> (element=w1314:bool)
      n654 = Index Array(array=w1333, index=5) -> (element=w1313:bool)
      n655 = Index Array(array=w1333, index=4) -> (element=w1312:bool)
      n656 = Index Array(array=w1333, index=3) -> (element=w1311:bool)
      n657 = Index Array(array=w1333, index=2) -> (element=w1310:bool)
      n658 = Index Array(array=w1333, index=1) -> (element=w1309:bool)
      n659 = Index Array(array=w1333, index=0) -> (element=w1308:bool)
    }
    n660 = node-c288(w1297) -> ()
  }
  n661 = while "Control APD data integration - stream to host" {
    shift-right: [w1390] -> _
    shift-left: w3 -> [w1395]
    stop <- FALSE stop-if-true
    n662 = flat-sequence {
      tunnel: w1395 -> [w1397]
      tunnel: [w1398] -> w1393
      tunnel: [w1397] -> w1391
      tunnel: [w1408] -> w1394
      tunnel: w1393 -> [w1408]
      tunnel: [w1407] -> w1392
      tunnel: w1391 -> [w1407]
      tunnel: [w1406] -> w1389
      tunnel: [w1405] -> w1388
      tunnel: [w1399] -> w1387
      tunnel: [w1451] -> w1390
      tunnel: w1394 -> [w1460]
      tunnel: w1392 -> [w1457]
      tunnel: w1389 -> [w1444]
      tunnel: w1388 -> [w1443]
      tunnel: w1387 -> [w1432]
      frame #0 {
        n663 = call "Loop Timer6"("Count(Ticks)"=w1397) -> ("Tick Count(Ticks)"=w1398:u32)
      }
      frame #1 {
        n664 = flat-sequence {
          tunnel: [w1410] -> w1404
          tunnel: w1404 -> [w1415]
          tunnel: [w1417] -> w1403
          tunnel: [w1416] -> w1402
          tunnel: [w1415] -> w1401
          tunnel: [i16 0] -> w1400
          tunnel: [w1424] -> w1405
          tunnel: [w1425] -> w1406
          tunnel: w1403 -> [w1425]
          tunnel: w1402 -> [w1424]
          tunnel: w1401 -> [w1423]
          tunnel: w1400 -> [w1422]
          tunnel: [w1422] -> w1399
          frame #0 {
            # "use separate variable so each APD won't\nhave to wait to read"
            n665 = feedback #56(FALSE) -> (w1409:bool)
            "APD1 out state" <- w1409
            "APD2 out state" <- w1409
            "APD3 out state" <- w1409
            n666 = Not(x=w1409) -> (.not. x?=w1410:bool)
            n667 = feedback-in #56(w1410) -> ()
          }
          frame #1 {
            n668 = local read "APD 3 Counts 1"() -> (w1413:u32)
            n669 = local read "APD 3 Counts 0"() -> (w1412:u32)
            n670 = local read "APD 1 Counts 1"() -> (w1421:u32)
            n671 = local read "APD 1 Counts 0"() -> (w1420:u32)
            n672 = local read "APD 2 Counts 1"() -> (w1419:u32)
            n673 = local read "APD 2 Counts 0"() -> (w1418:u32)
            n674 = Select(t=w1413, s=w1415, f=w1412) -> ()  [unwired: 1 out]
            n675 = Select(t=w1421, s=w1415, f=w1420) -> (s? t:f=w1417:u32)
            n676 = Select(t=w1419, s=w1415, f=w1418) -> (s? t:f=w1416:u32)
          }
          frame #2 {
            n677 = case shown="False" w1423 {
              frame False {
                w1426 = u32 0 ("APD 1 Counts 0")
                n678 = local write "APD 1 Counts 0"(w1426) -> ()
                n679 = local write "APD 2 Counts 0"(w1426) -> ()
                n680 = local write "APD 3 Counts 0"(w1426) -> ()
              }
              frame True {
                w1427 = u32 0 ("APD 1 Counts 1")
                n681 = local write "APD 1 Counts 1"(w1427) -> ()
                n682 = local write "APD 2 Counts 1"(w1427) -> ()
                n683 = local write "APD 3 Counts 1"(w1427) -> ()
              }
            }
          }
        }
      }
      frame #2 {
        # "crude initialization: if APD to FIFO is off (usually\nonly before initializing a measurement) count is forced to 0\nand green to true"
        # "count cycles till switching"
        n684 = feedback-in #57(w1460) -> ()
        n685 = feedback #57(w1460) -> (w1459:u32)
        n686 = Subtract(x=w1460, y=w1459) -> (x-y=w1458:u32)
        n687 = Subtract(x=w1458, y=w1457) -> (x-y=w1428:u32)
        n688 = case shown="True" "APD to FIFO" {
          tunnel: w1444 -> [_ w1465]
          tunnel: w1443 -> [_ w1463]
          tunnel: w1432 -> [_ w1461]
          frame False {
          }
          frame True {
            n689 = flat-sequence {
              tunnel: 0 ("Timeout") -> [w1467]
              tunnel: w1465 -> [w1468]
              tunnel: [w1467] -> w1464
              tunnel: w1464 -> [w1469]
              tunnel: w1463 -> [w1470]
              tunnel: [w1469] -> w1462
              tunnel: w1462 -> [w1472]
              tunnel: w1461 -> [w1471]
              frame #0 {
                n690 = xnode ("FIFO Write")("Element"=w1468, "Timeout"=w1467) -> ()  [unwired: 1 in, 2 out]
              }
              frame #1 {
                n691 = xnode ("FIFO Write")("Element"=w1470, "Timeout"=w1469) -> ()  [unwired: 1 in, 2 out]
              }
              frame #2 {
                n692 = xnode ("FIFO Write")("Element"=w1471, "Timeout"=w1472) -> ()  [unwired: 1 in, 2 out]
              }
            }
          }
        }
        n693 = Subtract(x="APD Acq Rate Count", y=w1428) -> (x-y=w1452:u32)
        n694 = Number To Boolean Array(number=w1428) -> (Boolean array=w1437:bool[])
        n695 = Or Array Elements(Boolean array=w1437) -> (logical OR=w1436:bool)
        n696 = Boolean To (0,1)(Boolean=w1436) -> (0, 1=w1442:i16)
        n697 = To Unsigned Byte Integer(number=w1442) -> (unsigned 8bit integer=w1439:u8)
        n698 = feedback #58(u8 0) -> (w1440:u8)
        n699 = Add(x=w1439, y=w1440) -> (x+y=w1438:u8)
        "APD Acq Late Counter" <- w1438
        n700 = feedback-in #58(w1438) -> ()
        n701 = Boolean To (0,1)(Boolean="+ phase (APD Acq)") -> (0, 1=w1448:i16)
        n702 = Multiply(x=w1448, y="Phase Count Adjustment (APD Acq)") -> (x*y=w1445:i16)
        n703 = Add(x=w1452, y=w1445) -> (x+y=w1451:u32)
        n704 = feedback #59(i16 0) -> (w1450:i16)
        n705 = Subtract(x=w1450, y=w1445) -> (x-y=w1447:i16)
        "APD Acq Relative Phase" <- w1447
        n706 = feedback-in #59(w1447) -> ()
        n707 = To Word Integer(number=w1444) -> (16bit integer=w1453:i16)
        n708 = To Word Integer(number=w1432) -> (16bit integer=w1433:i16)
        n709 = To Word Integer(number=w1443) -> (16bit integer=w1454:i16)
        n710 = Multiply(x="APD AO scale factor", y=w1454) -> (x*y=w1434:i16)
        n711 = Multiply(x="APD AO scale factor", y=w1433) -> (x*y=w1430:i16)
        n712 = Multiply(x="APD AO scale factor", y=w1453) -> (x*y=w1435:i16)
        n713 = xnode "FPGA I/O Node"("Connector0/AO5"=w1435, "Connector0/AO7"=w1434, "Connector0/AO6"=w1430) -> ()  [unwired: 3 in, 3 out]
      }
    }
  }
  n714 = while "APD 1 Gating" {
    shift-right: [w1476] -> _
    shift-left: w4 -> [w1481]
    shift-right: [w1475] -> _
    shift-left: w5 -> [w1473]
    stop <- FALSE stop-if-true
    n715 = flat-sequence {
      tunnel: w1481 -> [w1484]
      tunnel: [w1485] -> w1479
      tunnel: [w1484] -> w1477
      tunnel: [w1483] -> w1474
      tunnel: w1473 -> [w1483]
      tunnel: [w1488] -> w1480
      tunnel: w1479 -> [w1488]
      tunnel: [w1487] -> w1478
      tunnel: w1477 -> [w1487]
      tunnel: w1474 -> [w1486]
      tunnel: [w1506] -> w1476
      tunnel: w1480 -> [w1520]
      tunnel: w1478 -> [w1517]
      tunnel: [w1489] -> w1475
      frame #0 {
        n716 = call "Loop Timer7"("Count(Ticks)"=w1484) -> ("Tick Count(Ticks)"=w1485:u16)
      }
      frame #1 {
        # "Signal maybe then sent through \na transistor before APD"
        n717 = xnode "FPGA I/O Node"("Connector0/DIO0"=w1486) -> ()  [unwired: 1 in, 1 out]
        "APD1 int gate" <- w1486
      }
      frame #2 {
        n718 = feedback #60(TRUE) -> (w1512:bool)
        n719 = feedback-in #61(w1520) -> ()
        n720 = feedback #61(w1520) -> (w1519:u16)
        n721 = Not(x=w1512) -> (.not. x?=w1509:bool)
        n722 = feedback-in #60(w1509) -> ()
        n723 = Subtract(x=w1520, y=w1519) -> (x-y=w1518:u16)
        n724 = Select(t="APD Gate ON Count", s=w1509, f="APD Gate OFF Count") -> (s? t:f=w1514:u16)
        n725 = Subtract(x=w1518, y=w1517) -> (x-y=w1494:u16)
        n726 = Subtract(x=w1514, y=w1494) -> (x-y=w1505:u16)
        n727 = Number To Boolean Array(number=w1494) -> (Boolean array=w1495:bool[])
        n728 = Or Array Elements(Boolean array=w1495) -> (logical OR=w1493:bool)
        n729 = Boolean To (0,1)(Boolean="+ phase (APD 1 Gate)") -> (0, 1=w1503:i16)
        n730 = Boolean To (0,1)(Boolean=w1493) -> (0, 1=w1500:i16)
        n731 = Multiply(x=w1503, y="Phase count adjustment (APD 1 Gate)") -> (x*y=w1501:i16)
        n732 = To Unsigned Byte Integer(number=w1500) -> (unsigned 8bit integer=w1497:u8)
        n733 = Add(x=w1505, y=w1501) -> (x+y=w1506:u16)
        n734 = feedback #62(i16 0) -> (w1508:i16)
        n735 = Subtract(x=w1508, y=w1501) -> (x-y=w1507:i16)
        "APD 1 Gate Relative Phase" <- w1507
        n736 = feedback-in #62(w1507) -> ()
        n737 = feedback #63(u8 0) -> (w1498:u8)
        n738 = Add(x=w1497, y=w1498) -> (x+y=w1496:u8)
        "APD 1 Gate Late Counter" <- w1496
        n739 = feedback-in #63(w1496) -> ()
        n740 = case shown="2" "APD Gate Operating Mode" {
          tunnel: [TRUE FALSE w1523] -> w1490
          tunnel: w1512 -> [_ _ w1523]
          frame 0, Default {
          }
          frame 1 {
          }
          frame 2 {
          }
        }
        n741 = Not(x=w1490) -> (.not. x?=w1491:bool)
        n742 = Select(t=w1491, s="Invert APD Gate", f=w1490) -> (s? t:f=w1489:bool)
      }
    }
  }
  n743 = while "APD 2 Gating" {
    shift-right: [w1527] -> _
    shift-left: w4 -> [w1532]
    shift-right: [w1526] -> _
    shift-left: w5 -> [w1524]
    stop <- FALSE stop-if-true
    n744 = flat-sequence {
      tunnel: w1532 -> [w1535]
      tunnel: [w1536] -> w1530
      tunnel: [w1535] -> w1528
      tunnel: [w1534] -> w1525
      tunnel: w1524 -> [w1534]
      tunnel: [w1539] -> w1531
      tunnel: w1530 -> [w1539]
      tunnel: [w1538] -> w1529
      tunnel: w1528 -> [w1538]
      tunnel: w1525 -> [w1537]
      tunnel: [w1561] -> w1527
      tunnel: w1531 -> [w1571]
      tunnel: w1529 -> [w1569]
      tunnel: [w1540] -> w1526
      frame #0 {
        n745 = call "Loop Timer8"("Count(Ticks)"=w1535) -> ("Tick Count(Ticks)"=w1536:u16)
      }
      frame #1 {
        # "Signal maybe then sent through \na transistor before APD"
        n746 = xnode "FPGA I/O Node"("Connector0/DIO1"=w1537) -> ()  [unwired: 1 in, 1 out]
        "APD2 int gate" <- w1537
      }
      frame #2 {
        n747 = local read "APD Gate ON Count"() -> (w1554:u16)
        n748 = local read "APD Gate OFF Count"() -> (w1553:u16)
        n749 = feedback #64(TRUE) -> (w1566:bool)
        n750 = feedback-in #65(w1571) -> ()
        n751 = feedback #65(w1571) -> (w1555:u16)
        n752 = Not(x=w1566) -> (.not. x?=w1564:bool)
        n753 = feedback-in #64(w1564) -> ()
        n754 = Subtract(x=w1571, y=w1555) -> (x-y=w1570:u16)
        n755 = Select(t=w1554, s=w1564, f=w1553) -> (s? t:f=w1568:u16)
        n756 = Subtract(x=w1570, y=w1569) -> (x-y=w1546:u16)
        n757 = Subtract(x=w1568, y=w1546) -> (x-y=w1560:u16)
        n758 = Number To Boolean Array(number=w1546) -> (Boolean array=w1545:bool[])
        n759 = Or Array Elements(Boolean array=w1545) -> (logical OR=w1544:bool)
        n760 = Boolean To (0,1)(Boolean="+ phase (APD 2 Gate)") -> (0, 1=w1558:i16)
        n761 = Multiply(x=w1558, y="Phase count adjustment (APD 2 Gate)") -> (x*y=w1556:i16)
        n762 = Boolean To (0,1)(Boolean=w1544) -> (0, 1=w1551:i16)
        n763 = Add(x=w1560, y=w1556) -> (x+y=w1561:u16)
        n764 = To Unsigned Byte Integer(number=w1551) -> (unsigned 8bit integer=w1548:u8)
        n765 = feedback #66(i16 0) -> (w1563:i16)
        n766 = Subtract(x=w1563, y=w1556) -> (x-y=w1562:i16)
        "APD 2 Gate Relative Phase" <- w1562
        n767 = feedback-in #66(w1562) -> ()
        n768 = feedback #67(u8 0) -> (w1549:u8)
        n769 = Add(x=w1548, y=w1549) -> (x+y=w1547:u8)
        "APD 2 Gate Late Counter" <- w1547
        n770 = feedback-in #67(w1547) -> ()
        n771 = local read "APD Gate Operating Mode"() -> (w1552:u8)
        n772 = case shown="2" w1552 {
          tunnel: [TRUE FALSE w1574] -> w1541
          tunnel: w1566 -> [_ _ w1574]
          frame 0, Default {
          }
          frame 1 {
          }
          frame 2 {
          }
        }
        n773 = local read "Invert APD Gate"() -> (w1543:bool)
        n774 = Not(x=w1541) -> (.not. x?=w1542:bool)
        n775 = Select(t=w1542, s=w1543, f=w1541) -> (s? t:f=w1540:bool)
      }
    }
  }
  n776 = while "APD 3 Counter" {
    tunnel: w4 -> [_]
    stop <- FALSE stop-if-true
    n777 = flat-sequence {
      frame #0 {
        n778 = xnode "FPGA I/O Method Node"("FPGA I/O In"=refnum<k21> "Connector0/DIO12" ("APD 2 DO"), "Timeout"=-1) -> ()  [unwired: 2 out]
      }
      frame #1 {
        n779 = local read "APD3 int gate"() -> (w1578:bool)
        n780 = case shown="True" w1578 {
          frame False {
          }
          frame True {
            n781 = local read "APD3 out state"() -> (w1579:bool)
            n782 = case shown="True" w1579 {
              frame False {
                n783 = local read "APD 3 Counts 0"() -> (w1581:u32)
                n784 = Increment(x=w1581) -> (x+1=→"APD 3 Counts 0":u32)
              }
              frame True {
                n785 = local read "APD 3 Counts 1"() -> (w1583:u32)
                n786 = Increment(x=w1583) -> (x+1=→"APD 3 Counts 1":u32)
              }
            }
          }
        }
      }
    }
  }
  n787 = while "APD 3 Gating" {
    shift-right: [w1587] -> _
    shift-left: w4 -> [w1592]
    shift-right: [w1586] -> _
    shift-left: w5 -> [w1584]
    stop <- FALSE stop-if-true
    n788 = flat-sequence {
      tunnel: w1592 -> [w1595]
      tunnel: [w1596] -> w1590
      tunnel: [w1595] -> w1588
      tunnel: [w1594] -> w1585
      tunnel: w1584 -> [w1594]
      tunnel: [w1599] -> w1591
      tunnel: w1590 -> [w1599]
      tunnel: [w1598] -> w1589
      tunnel: w1588 -> [w1598]
      tunnel: w1585 -> [w1597]
      tunnel: [w1620] -> w1587
      tunnel: w1591 -> [w1631]
      tunnel: w1589 -> [w1628]
      tunnel: [w1600] -> w1586
      frame #0 {
        n789 = call "Loop Timer15"("Count(Ticks)"=w1595) -> ("Tick Count(Ticks)"=w1596:u16)
      }
      frame #1 {
        # "Signal maybe then sent through \na transistor before APD"
        n790 = xnode "FPGA I/O Node"("Connector0/DIO2"=w1597) -> ()  [unwired: 1 in, 1 out]
        "APD3 int gate" <- w1597
      }
      frame #2 {
        n791 = local read "APD Gate OFF Count"() -> (w1605:u16)
        n792 = local read "APD Gate ON Count"() -> (w1606:u16)
        n793 = feedback #68(TRUE) -> (w1625:bool)
        n794 = feedback-in #69(w1631) -> ()
        n795 = feedback #69(w1631) -> (w1630:u16)
        n796 = Not(x=w1625) -> (.not. x?=w1623:bool)
        n797 = feedback-in #68(w1623) -> ()
        n798 = Subtract(x=w1631, y=w1630) -> (x-y=w1629:u16)
        n799 = Select(t=w1606, s=w1623, f=w1605) -> (s? t:f=w1627:u16)
        n800 = Subtract(x=w1629, y=w1628) -> (x-y=w1608:u16)
        n801 = Subtract(x=w1627, y=w1608) -> (x-y=w1619:u16)
        n802 = Number To Boolean Array(number=w1608) -> (Boolean array=w1609:bool[])
        n803 = Or Array Elements(Boolean array=w1609) -> (logical OR=w1607:bool)
        n804 = Boolean To (0,1)(Boolean=w1607) -> (0, 1=w1614:i16)
        n805 = Boolean To (0,1)(Boolean="+ phase (APD 3 Gate)") -> (0, 1=w1617:i16)
        n806 = To Unsigned Byte Integer(number=w1614) -> (unsigned 8bit integer=w1611:u8)
        n807 = Multiply(x=w1617, y="Phase count adjustment (APD 3 Gate)") -> (x*y=w1615:i16)
        n808 = feedback #70(u8 0) -> (w1612:u8)
        n809 = Add(x=w1611, y=w1612) -> (x+y=w1610:u8)
        "APD 3 Gate Late Counter" <- w1610
        n810 = feedback-in #70(w1610) -> ()
        n811 = Add(x=w1619, y=w1615) -> (x+y=w1620:u16)
        n812 = feedback #71(i16 0) -> (w1622:i16)
        n813 = Subtract(x=w1622, y=w1615) -> (x-y=w1621:i16)
        "APD 3 Gate Relative Phase" <- w1621
        n814 = feedback-in #71(w1621) -> ()
        n815 = local read "APD Gate Operating Mode"() -> (w1604:u8)
        n816 = case shown="2" w1604 {
          tunnel: [TRUE FALSE w1634] -> w1601
          tunnel: w1625 -> [_ _ w1634]
          frame 0, Default {
          }
          frame 1 {
          }
          frame 2 {
          }
        }
        n817 = local read "Invert APD Gate"() -> (w1603:bool)
        n818 = Not(x=w1601) -> (.not. x?=w1602:bool)
        n819 = Select(t=w1602, s=w1603, f=w1601) -> (s? t:f=w1600:bool)
      }
    }
  }
  n820 = while {
    shift-right: [w1637] -> _
    shift-left: w4 -> [w1643]
    shift-right: [w1638] -> _
    shift-left: _ -> [w1635]
    stop <- FALSE stop-if-true
    n821 = flat-sequence {
      tunnel: w1643 -> [w1646]
      tunnel: [w1647] -> w1641
      tunnel: [w1646] -> w1639
      tunnel: [w1645] -> w1636
      tunnel: w1635 -> [w1645]
      tunnel: [w1650] -> w1642
      tunnel: w1641 -> [w1650]
      tunnel: [w1649] -> w1640
      tunnel: w1639 -> [w1649]
      tunnel: w1636 -> [w1648]
      tunnel: w1642 -> [w1680]
      tunnel: w1640 -> [w1679]
      tunnel: [w1652] -> w1638
      tunnel: [w1651] -> w1637
      frame #0 {
        n822 = call "Loop Timer2"("Count(Ticks)"=w1646) -> ("Tick Count(Ticks)"=w1647:u16)
      }
      frame #1 {
        n823 = xnode "FPGA I/O Node"("Connector0/DIO10"=w1648) -> ()  [unwired: 1 in, 1 out]
      }
      frame #2 {
        n824 = feedback #72(w1680) -> (w1681:u16)
        n825 = feedback-in #72(w1680) -> ()
        n826 = Subtract(x=w1680, y=w1681) -> (x-y=w1682:u16)
        n827 = Subtract(x=w1682, y=w1679) -> (x-y=w1672:u16)
        n828 = Number To Boolean Array(number=w1672) -> (Boolean array=w1677:bool[])
        n829 = Or Array Elements(Boolean array=w1677) -> (logical OR=w1678:bool)
        n830 = Boolean To (0,1)(Boolean="+ phase (EMCCD Gate)") -> (0, 1=w1665:i16)
        n831 = Boolean To (0,1)(Boolean=w1678) -> (0, 1=w1673:i16)
        n832 = To Unsigned Byte Integer(number=w1673) -> (unsigned 8bit integer=w1676:u8)
        n833 = Multiply(x=w1665, y="Phase Count Adjustment EMCCD Gate") -> (x*y=w1667:i16)
        n834 = feedback #73(u8 0) -> (w1675:u8)
        n835 = Add(x=w1676, y=w1675) -> (x+y=w1671:u8)
        "EMCCD Late counter" <- w1671
        n836 = feedback-in #73(w1671) -> ()
        n837 = feedback #74(i16 0) -> (w1666:i16)
        n838 = Subtract(x=w1666, y=w1667) -> (x-y=w1660:i16)
        "EMCCD relative phase" <- w1660
        n839 = feedback-in #74(w1660) -> ()
        n840 = feedback #75(TRUE) -> (w1658:bool)
        n841 = Not(x=w1658) -> (.not. x?=w1656:bool)
        n842 = Select(t="EMCCD Gate ON count", s=w1656, f="EMCCD Gate OFF count") -> (s? t:f=w1668:u16)
        n843 = Subtract(x=w1668, y=w1672) -> (x-y=w1661:u16)
        n844 = Add(x=w1661, y=w1667) -> (x+y=w1651:u16)
        n845 = feedback-in #75(w1656) -> ()
        n846 = case shown="1" "EMCCD Gate Operating Mode" {
          tunnel: w1656 -> [_ _ w1685]
          tunnel: [TRUE FALSE w1685] -> w1654
          frame 0, Default {
          }
          frame 1 {
          }
          frame 2 {
          }
        }
        n847 = Not(x=w1654) -> (.not. x?=w1655:bool)
        n848 = Select(t=w1655, s="Invert EMCCD Gate", f=w1654) -> (s? t:f=w1652:bool)
      }
    }
  }
  n849 = disable-structure shown="Disabled" {
    disable-tunnel: w4 -> [w1688 _]
    disable-tunnel: w15 -> [w1687 _]
    frame Disabled {
      n850 = while "633 nm red  fluorescent laser interlacing (DO to IA 633 nm AOM ME amp)." {
        shift-right: [w1809] -> _
        shift-left: w1688 -> [w1814]
        shift-right: [w1808] -> _
        shift-left: w1687 -> [w1806]
        stop <- FALSE stop-if-true
        n851 = flat-sequence {
          tunnel: w1814 -> [w1817]
          tunnel: [w1818] -> w1812
          tunnel: [w1817] -> w1810
          tunnel: [w1816] -> w1807
          tunnel: w1806 -> [w1816]
          tunnel: [w1821] -> w1813
          tunnel: w1812 -> [w1821]
          tunnel: [w1820] -> w1811
          tunnel: w1810 -> [w1820]
          tunnel: w1807 -> [w1819]
          tunnel: [w1830] -> w1809
          tunnel: w1813 -> [w1850]
          tunnel: w1811 -> [w1847]
          tunnel: [w1839] -> w1808
          frame #0 {
            n852 = call "Loop Timer11"("Count(Ticks)"=w1817) -> ("Tick Count(Ticks)"=w1818:u16)
          }
          frame #1 {
            # "Then to PRL 440 amp"
            n853 = xnode "FPGA I/O Node"("Connector1/DIO32"=w1819) -> ()  [unwired: 1 in, 1 out]
          }
          frame #2 {
            n854 = feedback-in #76(w1850) -> ()
            n855 = feedback #76(w1850) -> (w1849:u16)
            n856 = Subtract(x=w1850, y=w1849) -> (x-y=w1848:u16)
            n857 = Subtract(x=w1848, y=w1847) -> (x-y=w1823:u16)
            n858 = Number To Boolean Array(number=w1823) -> (Boolean array=w1824:bool[])
            n859 = Or Array Elements(Boolean array=w1824) -> (logical OR=w1822:bool)
            n860 = Boolean To (0,1)(Boolean="+ phase (RI)") -> (0, 1=w1835:i16)
            n861 = Multiply(x=w1835, y="Phase count adjustment (RI)") -> (x*y=w1832:i16)
            n862 = Boolean To (0,1)(Boolean=w1822) -> (0, 1=w1829:i16)
            n863 = To Unsigned Byte Integer(number=w1829) -> (unsigned 8bit integer=w1826:u8)
            n864 = feedback #77(i16 0) -> (w1833:i16)
            n865 = feedback #78(u8 0) -> (w1827:u8)
            n866 = Add(x=w1826, y=w1827) -> (x+y=w1825:u8)
            "RI Late Counter" <- w1825
            n867 = feedback-in #78(w1825) -> ()
            n868 = Subtract(x=w1833, y=w1832) -> (x-y=w1831:i16)
            "RI Relative phase" <- w1831
            n869 = feedback-in #77(w1831) -> ()
            n870 = feedback #79(TRUE) -> (w1842:bool)
            n871 = case shown="2" "Red Laser Operating Mode" {
              tunnel: [TRUE FALSE w1856] -> w1839
              tunnel: w1842 -> [_ _ w1853]
              frame 0, Default {
              }
              frame 1 {
              }
              frame 2 {
                n872 = Not(x=w1853) -> (.not. x?=w1855:bool)
                n873 = Select(t=w1855, s="Invert RI", f=w1853) -> (s? t:f=w1856:bool)
              }
            }
            n874 = Not(x=w1842) -> (.not. x?=w1838:bool)
            n875 = Select(t="Red interlace ON count", s=w1838, f="Red interlace OFF count") -> (s? t:f=w1844:u16)
            n876 = Subtract(x=w1844, y=w1823) -> (x-y=w1836:u16)
            n877 = Add(x=w1836, y=w1832) -> (x+y=w1830:u16)
            n878 = feedback-in #79(w1838) -> ()
          }
        }
      }
      n879 = while "473 nm blue  fluorescent laser interlacing (DO to blue laser digital control input)." {
        shift-right: [w1705] -> _
        shift-left: w1688 -> [w1708]
        shift-right: [w1704] -> _
        shift-left: w1687 -> [w1702]
        shift-right: [w1697] -> _
        shift-left: _ -> [w1696]
        shift-right: [w1689] -> _
        shift-left: u16 0 -> [w1692]
        stop <- FALSE stop-if-true
        n880 = flat-sequence {
          tunnel: w1708 -> [w1713]
          tunnel: [w1714] -> w1707
          tunnel: [w1713] -> w1706
          tunnel: [w1712] -> w1703
          tunnel: w1702 -> [w1712]
          tunnel: w1696 -> [w1711]
          tunnel: [w1711] -> w1695
          tunnel: [w1710] -> w1693
          tunnel: w1692 -> [w1710]
          tunnel: [w1719] -> w1701
          tunnel: w1707 -> [w1719]
          tunnel: [w1718] -> w1700
          tunnel: w1706 -> [w1718]
          tunnel: w1703 -> [w1717]
          tunnel: w1695 -> [w1716]
          tunnel: [w1716] -> w1694
          tunnel: w1693 -> [w1715]
          tunnel: [w1715] -> w1691
          tunnel: [w1724] -> w1699
          tunnel: [w1723] -> w1698
          tunnel: w1700 -> [w1723]
          tunnel: w1701 -> [w1724]
          tunnel: w1694 -> [w1722]
          tunnel: w1691 -> [w1721]
          tunnel: [w1720] -> w1690
          tunnel: [w1781] -> w1705
          tunnel: w1699 -> [w1799]
          tunnel: w1698 -> [w1796]
          tunnel: [w1769] -> w1704
          tunnel: [w1767] -> w1697
          tunnel: w1690 -> [w1764]
          tunnel: [w1765] -> w1689
          frame #0 {
            n881 = call "Loop Timer14"("Count(Ticks)"=w1713) -> ("Tick Count(Ticks)"=w1714:u16)
          }
          frame #1 {
            n882 = xnode "FPGA I/O Node"("Connector1/DIO28"=w1717) -> ()  [unwired: 1 in, 1 out]
          }
          frame #2 {
            n883 = case shown="True" w1722 {
              tunnel: w1721 -> [w1725 w1727]
              tunnel: [w1725 w1726] -> w1720
              frame False {
              }
              frame True {
                n884 = flat-sequence {
                  tunnel: [w1733] -> w1730
                  tunnel: [w1732] -> w1729
                  tunnel: [w1731] -> w1728
                  tunnel: w1727 -> [w1731]
                  tunnel: w1730 -> [w1750]
                  tunnel: w1729 -> [w1747]
                  tunnel: w1728 -> [w1749]
                  tunnel: [w1748] -> w1726
                  frame #0 {
                    # "5 ns timing resolution"
                    n885 = node-c288() -> (w1736:T6)  [unwired: 1 in]
                    n886 = timed-loop {
                      timing: w1736 -> [_]
                      timing-out: [_] -> w1735
                      tunnel: "Lifetime timeout APD1" -> [w1742]
                      tunnel: [w1737] -> w1732
                      tunnel: [w1738] -> w1733
                      i -> [w1739]
                      stop <- w1741 stop-if-true
                      n887 = xnode "FPGA I/O Node"() -> ("Connector0/DIO5"=w1740:bool)  [unwired: 1 in, 1 out]
                      n888 = To Unsigned Word Integer(number=w1739) -> (unsigned 16bit integer=w1737:u16)
                      n889 = Equal?(x=w1742, y=w1737) -> (x = y?=w1738:bool)
                      n890 = Or(x=w1740, y=w1738) -> (x .or. y?=w1741:bool)
                    }
                    n891 = node-c288(w1735) -> ()
                  }
                  frame #1 {
                    n892 = Not(x=w1750) -> (.not. x?=w1751:bool)
                    n893 = case shown="True" w1751 {
                      tunnel: w1747 -> [_ w1753]
                      tunnel: w1749 -> [w1752 w1755]
                      tunnel: [w1752 w1754] -> w1748
                      frame False {
                        # "timed out, do nothing"
                      }
                      frame True {
                        # "photon detected,record time"
                        n894 = case shown="True" "Lifetime to FIFO" {
                          tunnel: w1753 -> [_ w1761]
                          tunnel: w1755 -> [w1757 w1759]
                          tunnel: [w1757 w1758] -> w1754
                          frame False {
                            # "don't record time\n(can't if doing force feedback)"
                          }
                          frame True {
                            # "number of events in fifo"
                            n895 = xnode ("FIFO Method Node")("Element"=w1761, "Timeout"=0) -> ()  [unwired: 1 in, 2 out]
                            n896 = Increment(x=w1759) -> (x+1=w1758:u16)
                          }
                        }
                        "lifetime (ticks)" <- w1753
                      }
                    }
                  }
                }
              }
            }
          }
          frame #3 {
            # "Reading fifo is tricky here since\nunknown # of events"
            # "For lifetime measurement:\nInterlacing and pulse falling"
            n897 = feedback-in #80(w1799) -> ()
            n898 = feedback #80(w1799) -> (w1798:u16)
            n899 = Subtract(x=w1799, y=w1798) -> (x-y=w1797:u16)
            n900 = Subtract(x=w1797, y=w1796) -> (x-y=w1774:u16)
            n901 = Number To Boolean Array(number=w1774) -> (Boolean array=w1775:bool[])
            n902 = Or Array Elements(Boolean array=w1775) -> (logical OR=w1773:bool)
            n903 = Boolean To (0,1)(Boolean="+ phase (BI D)") -> (0, 1=w1786:i16)
            n904 = Multiply(x=w1786, y="Phase count adjustment (BI D)") -> (x*y=w1783:i16)
            n905 = Boolean To (0,1)(Boolean=w1773) -> (0, 1=w1780:i16)
            n906 = To Unsigned Byte Integer(number=w1780) -> (unsigned 8bit integer=w1777:u8)
            n907 = feedback #81(i16 0) -> (w1784:i16)
            n908 = feedback #82(u8 0) -> (w1778:u8)
            n909 = Add(x=w1777, y=w1778) -> (x+y=w1776:u8)
            "Blue Late Counter (D)" <- w1776
            n910 = feedback-in #82(w1776) -> ()
            n911 = Subtract(x=w1784, y=w1783) -> (x-y=w1782:i16)
            "BI Relative phase (D)" <- w1782
            n912 = feedback-in #81(w1782) -> ()
            n913 = feedback #83(TRUE) -> (w1791:bool)
            n914 = case shown="2" "Blue Laser Operating Mode (D)" {
              tunnel: [TRUE FALSE w1805] -> w1769
              tunnel: w1791 -> [_ _ w1802]
              frame 0, Default {
              }
              frame 1 {
              }
              frame 2 {
                n915 = Not(x=w1802) -> (.not. x?=w1804:bool)
                n916 = Select(t=w1804, s="Invert BI (D)", f=w1802) -> (s? t:f=w1805:bool)
              }
            }
            n917 = Subtract(x=w1764, y="Lifetime events to read blue") -> (x-y=w1762:u16)
            n918 = Not(x=w1791) -> (.not. x?=w1789:bool)
            n919 = Select(t="Blue interlace ON count (D)", s=w1789, f="Blue interlace OFF count (D)") -> (s? t:f=w1793:u16)
            n920 = Subtract(x=w1793, y=w1774) -> (x-y=w1787:u16)
            n921 = Add(x=w1787, y=w1783) -> (x+y=w1781:u16)
            n922 = feedback-in #83(w1789) -> ()
            n923 = Select(t=w1762, s="Lifetime read blue fifo", f=w1764) -> (s? t:f=w1765:u16)
            "lifetime events in fifo" <- w1765
            n924 = Equal?(x="Blue Laser Operating Mode (D)", y=u8 2) -> (x = y?=w1770:bool)
            n925 = Not(x=w1769) -> (.not. x?=w1768:bool)
            n926 = And(x=w1768, y=w1770) -> (x .and. y?=w1767:bool)
          }
        }
      }
    }
    frame Enabled {
    }
  }
